vi "Trajectory Builder.vi"() -> ()   [LabVIEW 2019]
uses:
  Limits.ctl
  Command Stuff/Command Editor Info.ctl
  Command Stuff/Single Cmd Info.ctl
  <vilib>/picture/picture.llb/imagedata.ctl
  <vilib>/Utility/miscctls.llb/LVPositionTypeDef.ctl
  <vilib>/Utility/miscctls.llb/LVBoundsTypeDef.ctl
  Command Stuff/Availible Command systems for auto.ctl
  <vilib>/event_ctls.llb/lveventtype.ctl
  Globals.vi
panel:
  out "IRR":bool
  out "Trajectory Data":T1(array[cluster])
  in  "Reverse Path":bool
  in  "Robot Backwards":bool
  out "Picture":picture
  out "Duration (s)":dbl format="%#.4g"
  out "Distance (ft)":dbl format="%#.1g"
  in  "Instructions":string="Directions:\nUse mouse to ...\n    move robot position (rectangle with arrow)\n    rotate robot (red arrow)\n    move waypoints (numbered circles)\nClick in open space to add a waypoint\nShift click to delete a waypoint\nHover over a waypoint and use arrow keys to nudge\n\nTime slider and Play button will run robot along path to test for collisions.\n\nDirection and Destionation are folder selectors for files\n\nNew creates a new path at default location\n\nAppend creates a path using current path's position and heading.\n\nTo add a command, move robot using Time slider and double click Command in Palette.\n\nYou can modify command timing in the graph or Command Sequencer tree.\n\nEnable/disable a command by clicking on the enable column item.\n\nDelete a command by shift-clicking in the enable column.\n\nTo configure command parameters, Select the command name in the tree, Open Panel, enter parameters, and Inhale the parameters."
  out "WayPoints":cluster{"x":dbl, "y":dbl, "th":dbl}[](array[cluster]) {"th" format="%#_4g"}
  in  "Scale Factor":dbl=0.75
  out "Command Palette":picture
  in  "Cache":T5
  out "folder names":cluster{"name":string, "name":string}
  in  "Directory":bool
  in  "Tab Control":T6(tab)
  in  "Overrides":T7(array[cluster]) {"Angular Multiplier 2" step=5.0; "Angular Multiplier" step=5.0}
  in  "Allow Angles > 90":bool
  in  "Stoopid Overlap %":dbl min=0.0
  in  "Center Flip":bool
  in  "Snap to foot":bool
  in  "Angle Limiter":enum16{"90", "45", "15", "1"}(ring)=enum."15"
  in  "Snap robot to baseline":bool
  in  "Sample Period (s)":dbl=0.02 format="%#_6p"
  in  "Limits":T8={"Velocity (fps)"=6.0, "Accel (fps^2)"=15.0, "Jerk (fps^3)"=150.0, "StoopidFast (fps)"=6.0} {"StoopidFast (fps)" min=0.0; "Jerk (fps^3)" min=0.0 step=1.0; "Accel (fps^2)" min=0.0; "Velocity (fps)" min=0.0}
  in  "Conditions":T9 {"vFinal (fps)" min=0.0; "vInitial (fps)" min=0.0}
  in  "Unjank":bool
  in  "Turn Acceleration":bool=TRUE
  in  "Turn Deceleration":bool=TRUE
  in  "Hide Path":bool
  in  "Open Command":bool
  in  "Inhale":bool
  in  "Command Sequence":string(tree)
  in  "Projects":u16(ring) items=["2021 Robot.lvproj"]
  in  "Refresh":bool
  in  "Background":u16(ring) items=["IR Field", "Barrels", "Bounce", "Slalom", "Galactic Search A", "Galactic Search B"]
  in  "Robot Color":u32(colorbox)=14421504
  out "Field Size (ft)":cluster{"width":dbl, "height":dbl}={"width"=26.9167, "height"=35.2142} {"width" format="%#.1g"; "height" format="%#.1g"}
  in  "Robot Size (in)":cluster{"width":dbl, "height":dbl}={"width"=36.5, "height"=34.5}
  in  "Time (s)":dbl(slide) scale=0.0..3.62 scale format="%#.1g"
  in  "Play":bool
  in  "Sub Dir 2":u16(ring)
  in  "Sub Dir 1":u16(ring)
  out "fps":dbl[](graph)
  in  "Append":bool
  in  "Open":i32(listbox)
  in  "Filename":string
  in  "Save":bool
  in  "New":bool
  out "slalom":bool
  out "barrels":bool
  out "bounce":bool
  out "G-S B":bool
  out "G-S A":bool
  # "Command Palette"
  # "StupidFast makes each linear segment into a\nvelocity ramp to max speed"
  # "Nicotine"
  # "Interaction Options"
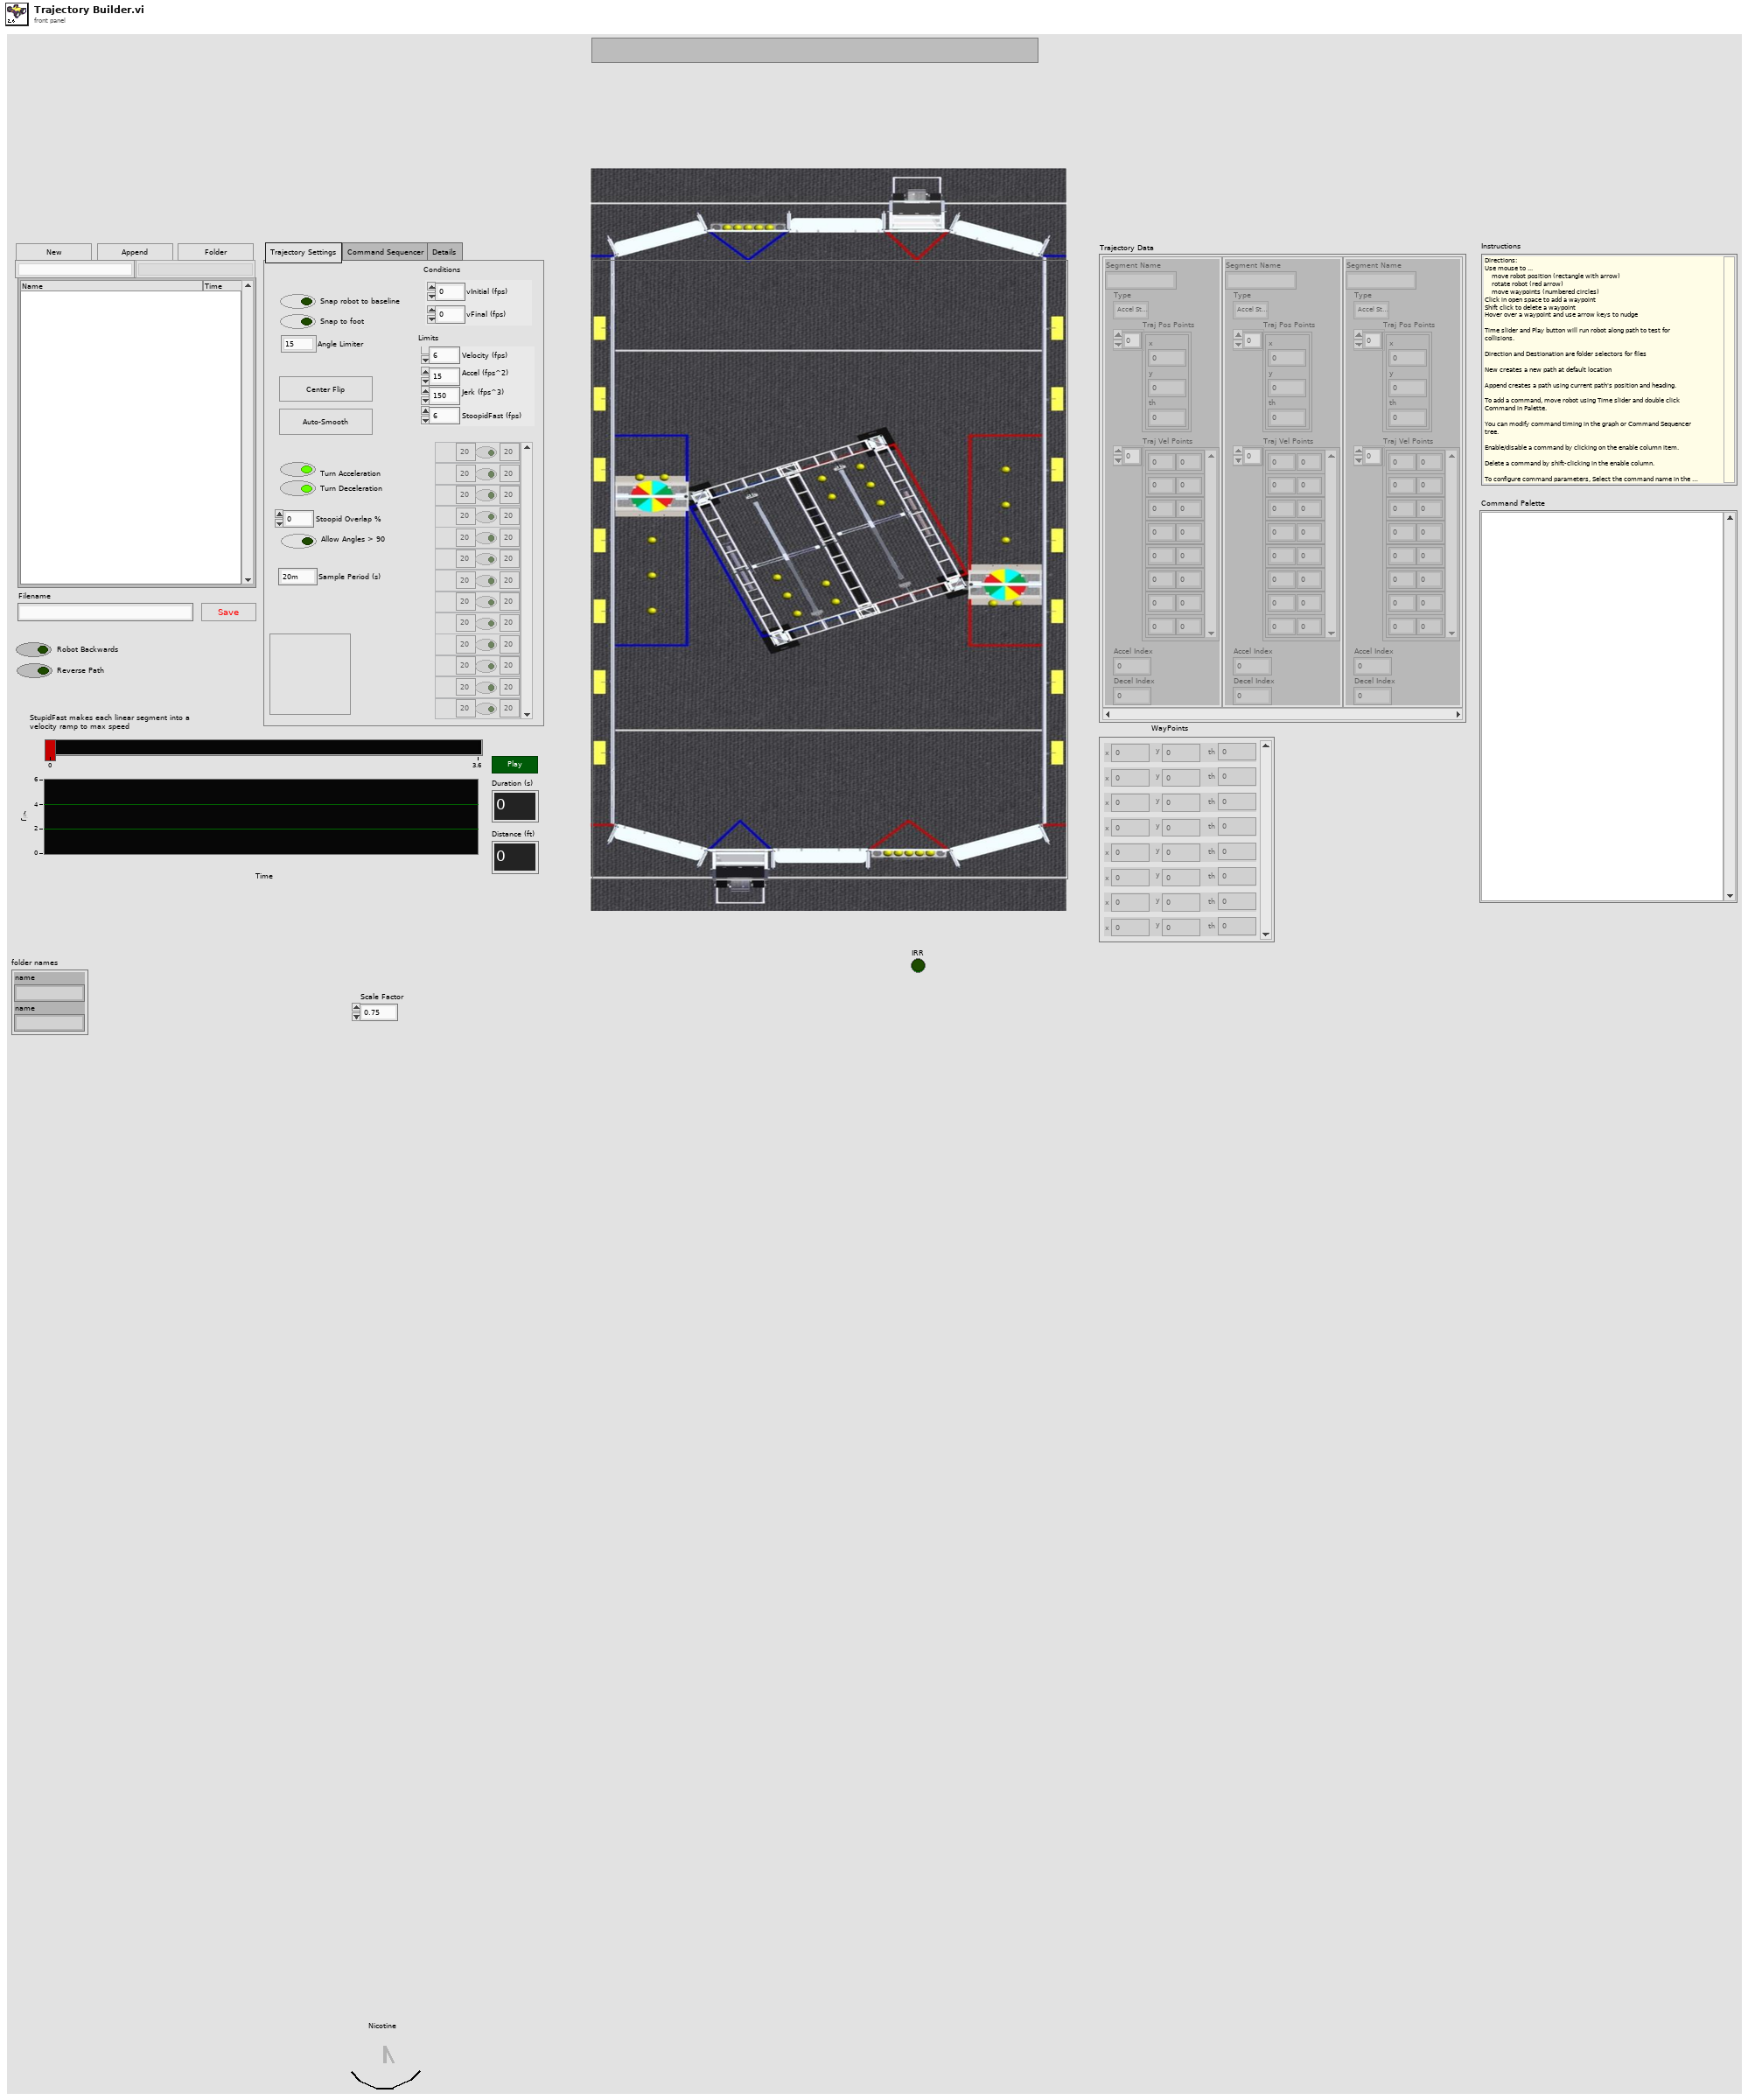
[diagram p1: front panel]
types:
  T1 = cluster{"Segment Name":string, "Type":enum16{"Accel Straight", "Const Straight", "Blend", "Circle"}, "Traj Pos Points":cluster{"x":dbl, "y":dbl, "th":dbl}[], "Traj Vel Points":cluster{"V":dbl, "th":dbl}[], "Accel Index":i32, "Decel Index":i32}[]
  T2 = typedef "Command Editor Info.ctl" = T3[]
  T3 = typedef "Single Cmd Info.ctl" = cluster{"Name":string, "CPTM.DataType":variant, "All Control Values Variant":cluster{"Name":string, "Variant Data":variant}[], "icon full":T4, "icon scaled":T4, "Path":path, "Subsystem Color":u32}
  T4 = typedef "imagedata.ctl" = cluster{"image type":i32, "image depth":i32, "image":u8[], "mask":u8[], "colors":u32[], "Rectangle":cluster{"left":i16, "top":i16, "right":i16, "bottom":i16}}
  T5 = cluster{"Filtered Command Info Out":T2, "2D Picture":picture}
  T6 = enum32{"Trajectory Settings", "Command Sequencer", "Details"}
  T7 = cluster{"Count":string, "Angular Multiplier":dbl, "1":bool, "Angular Multiplier 2":dbl}[]
  T8 = typedef "Limits.ctl" = cluster{"Velocity (fps)":dbl, "Accel (fps^2)":dbl, "Jerk (fps^3)":dbl, "StoopidFast (fps)":dbl}
  T9 = cluster{"vInitial (fps)":dbl, "vFinal (fps)":dbl}
  T10 = cluster{"Sample Period (s)":dbl, "Limits 2":T8, "Conditions":cluster{"vInitial (fps)":dbl, "vFinal (fps)":dbl}, "Angular \nAccelerations":cluster{string, "Angular Multiplier":dbl, "1":bool, "Angular Multiplier 2":dbl}[]}
  T11 = cluster{string, "Angular Multiplier":dbl, "1":bool, "Angular Multiplier 2":dbl}[]
  T12 = typedef "LVPositionTypeDef.ctl" = cluster{"Left":i32, "Top":i32}
  T13 = enum32{"Trajectory Settings", "Command Sequencer"}
  T14 = cluster{"Index":i32, "Pt Test Results":enum16{"Miss", "Rect Hit", "Arrow Hit"}}
  T15 = cluster{"Drag Object":cluster{"Index":i32, "x":dbl, "y":dbl}, "Hover Object":cluster{"Index":i32, "Pt Test Results":enum16{"Miss", "Rect Hit", "Arrow Hit"}}, "Filename":string}
  T16 = cluster{"Trajectory Data":cluster{"Segment Name":string, "Type":enum16{"Accel Straight", "Const Straight", "Blend", "Circle"}, "Traj Pos Points":cluster{"x":dbl, "y":dbl, "th":dbl}[], "Traj Vel Points":cluster{"V":dbl, "th":dbl}[], "Accel Index":i32, "Decel Index":i32}[], "Points":cluster{"x":dbl, "y":dbl, "th":dbl}[], "Cluster 2":cluster{"Sample Period (s)":dbl, "Limits 2":T8, "Conditions":cluster{"vInitial (fps)":dbl, "vFinal (fps)":dbl}, "Angular \nAccelerations":cluster{string, "Angular Multiplier":dbl, "1":bool, "Angular Multiplier 2":dbl}[]}, cluster{"Time (s)":dbl, T3, bool}[]}
  T17 = cluster{"Sample Period (s)":dbl, "Limits":cluster{"Velocity (fps)":dbl, "Accel (fps^2)":dbl, "Turn Accel (fps^2)":dbl, "Jerk (fps^3)":dbl}, "Conditions":cluster{"vInitial (fps)":dbl, "vFinal (fps)":dbl}, cluster{dbl[], bool[]}}
  T18 = cluster{"Sample Period (s)":dbl, "Limits":cluster{"Velocity (fps)":dbl, "Accel (fps^2)":dbl, "Jerk (fps^3)":dbl}, "Conditions":cluster{"vInitial (fps)":dbl, "vFinal (fps)":dbl}, " Acceleration Overrides":cluster{"Angular \nAccelerations":dbl[], "Accel Override Bools":bool[]}}
  T19 = typedef "LVBoundsTypeDef.ctl" = cluster{"Width":u32, "Height":u32}
  T20 = cluster{"Velocity":dbl, "Sample Time":dbl, "Accel":dbl}
  T21 = cluster{"Sample Period (s)":dbl, "Limits":cluster{"Velocity (fps)":dbl, "Acceleration (fps^2)":dbl, "Jerk (fps^3)":dbl}, "Conditions":cluster{"vInitial (fps)":dbl, "vFinal (fps)":dbl}}
  T22 = cluster{"Reverse Path":bool, "Robot Backwards":bool}
  T23 = cluster{"Sample Period (s)":dbl, "Limits 2":cluster{"Velocity (fps)":dbl, "Acceleration (fps^2)":dbl, "Jerk (fps^3)":dbl}, "Conditions":cluster{"vInitial (fps)":dbl, "vFinal (fps)":dbl}, " Acceleration Overrides":cluster{"Angular \nAccelerations":dbl[], "Accel Override Bools":bool[]}}
  T24 = cluster{"Sample Period (s)":dbl, "Limits":cluster{"Velocity (fps)":dbl, "Acceleration (fps^2)":dbl, "Jerk (fps^3)":dbl}, "Conditions":cluster{"vInitial (fps)":dbl, "vFinal (fps)":dbl}, "Min Rads":dbl[]}
  T25 = typedef "Availible Command systems for auto.ctl" = u16
  T26 = cluster{"Time into Path":dbl, "System":T25, "Item Selected?":bool, "System Selection":T25}[]
  T27 = cluster{"Sample Period (s)":dbl, "Limits 2":cluster{"Velocity (fps)":dbl, "Acceleration (fps^2)":dbl, "Jerk (fps^3)":dbl, "Stoopid Fast":dbl}, "Conditions":cluster{"vInitial (fps)":dbl, "vFinal (fps)":dbl}, " Acceleration Overrides":cluster{"Angular \nAccelerations":dbl[], "Accel Override Bools":bool[]}}
  T28 = typedef "lveventtype.ctl" = enum32{"Null", "Timeout", "Annotation Menu Selection", "Annotation Menu Selection?", "App Instance Close", "App Instance Close?", "Autoscale Range Change", "Bookmark Info Change", "Cell Edit", "Cell Edit?", "Cursor Grab", "Cursor Grab?", "Cursor Menu Selection", "Cursor Menu Selection?", "Cursor Move", "Cursor Release", "Data Change", "Direction Change", "Display State Change", "Drag Ended", "Drag Enter", "Drag Leave", "Drag Over", "Drag Source Update", "Drag Starting", "Drag Starting?", "Drop", "Exec State Change", "Key Down", "Key Down?", "Key Repeat", "Key Repeat?", "Key Up", "Listbox Double Click", "Menu Activation?", "Menu Selection (App)", "Menu Selection? (App)", "Menu Selection (User)", "Mouse Down", "Mouse Down?", "Mouse Enter", "Mouse Leave", "Mouse Move", "Mouse Up", "Mouse Wheel", "NI Security User Change (App)", "Pane Size", "Panel Close", "Panel Close?", "Panel Resize", "Plot Attribute Change", "Scale Range Change", "Shortcut Menu Activation?", "Shortcut Menu Selection (App)", "Shortcut Menu Selection? (App)", "Shortcut Menu Selection (User)", "Tree Double Click", "Tree Drag", "Tree Drag?", "Tree Drop", "Tree Drop?", "Tree Item Close", "Tree Item Close?", "Tree Item Open", "Tree Item Open?", "User Event", "Value Change"}
  T29 = enum32{"Invalid", "Standard", "Closed", "Hidden", "Minimized", "Maximized"}
  T30 = cluster{"Sample Period (s)":dbl, "Limits":T8, "Conditions":cluster{"vInitial (fps)":dbl, "vFinal (fps)":dbl}, "Overrides":cluster{"Count":string, "Angular Multiplier":dbl, "1":bool, "Angular Multiplier 2":dbl}[]}
  T31 = cluster{"width":dbl, "height":dbl, "width":dbl, "height":dbl}
  T32 = cluster{"Robot Backwards":bool, "Reverse Path":bool}
  T33 = cluster{"Sample Period (s)":dbl, "Limits":T8, "Conditions":cluster{"vInitial (fps)":dbl, "vFinal (fps)":dbl}, cluster{dbl[], bool[]}}
  T34 = cluster{"Trajectory Data":cluster{"Segment Name":string, "Type":enum16{"Accel Straight", "Const Straight", "Blend", "Circle"}, "Traj Pos Points":cluster{"x":dbl, "y":dbl, "th":dbl}[], "Traj Vel Points":cluster{"V":dbl, "th":dbl}[], "Accel Index":i32, "Decel Index":i32}[], "Updated Waypoints":cluster{"x":dbl, "y":dbl, "th":dbl}[], "Cluster 2":cluster{"Sample Period (s)":dbl, "Limits":T8, "Conditions":cluster{"vInitial (fps)":dbl, "vFinal (fps)":dbl}, "Overrides":cluster{"Count":string, "Angular Multiplier":dbl, "1":bool, "Angular Multiplier 2":dbl}[]}, cluster{"Time (s)":dbl, T3, bool}[]}
  T35 = cluster{"Velocity":dbl, "Accel":dbl, "Accel":dbl, "Velocity":dbl}
  T36 = cluster{"Velocity (fps)":dbl, "Acceleration (fps^2)":dbl, "Jerk (fps^3)":dbl}
  T37 = cluster{"Velocity (fps)":dbl, "Acceleration (fps^2)":dbl, "Jerk (fps^3)":dbl, "Velocity (fps)":dbl}
  T38 = cluster{string, "Angular Multiplier":dbl, bool, "Velocity (fps)":dbl}
  T39 = cluster{"Angular \nAccelerations":dbl[], "Accel Override Bools":bool[]}
  T40 = cluster{string, "Turn Accel":dbl, "Overtide":bool, "Velocity (fps)":dbl}[]
  T41 = cluster{"Velocity (fps)":dbl, "Acceleration (fps^2)":dbl, "Jerk (fps^3)":dbl, "Stoopid Fast":dbl}
  T42 = cluster{"Velocity (fps)":dbl, "Accel (fps^2)":dbl, "Turn Accel (fps^2)":dbl, "Jerk (fps^3)":dbl}
  T43 = cluster{"Sample Period (s)":dbl, cluster{"Velocity (fps)":dbl, "Accel (fps^2)":dbl, "Turn Accel (fps^2)":dbl, "Jerk (fps^3)":dbl}, "Conditions":cluster{"vInitial (fps)":dbl, "vFinal (fps)":dbl}, "Array":cluster{"Count":string, "Turn Accel":dbl, "Overtide":bool, "Velocity (fps)":dbl}[]}
  T44 = cluster{"Trajectory Data":cluster{"Segment Name":string, "Type":enum16{"Accel Straight", "Const Straight", "Blend", "Circle"}, "Traj Pos Points":cluster{"x":dbl, "y":dbl, "th":dbl}[], "Traj Vel Points":cluster{"V":dbl, "th":dbl}[], "Accel Index":i32, "Decel Index":i32}[], "Points":cluster{"x":dbl, "y":dbl, "th":dbl}[], cluster{"Sample Period (s)":dbl, cluster{"Velocity (fps)":dbl, "Accel (fps^2)":dbl, "Turn Accel (fps^2)":dbl, "Jerk (fps^3)":dbl}, "Conditions":cluster{"vInitial (fps)":dbl, "vFinal (fps)":dbl}, "Array":cluster{"Count":string, "Turn Accel":dbl, "Overtide":bool, "Velocity (fps)":dbl}[]}, cluster{"Time (s)":dbl, T3, bool}[]}
  T45 = typedef "LVPoint32TypeDef.ctl" = cluster{"Horizontal":i32, "Vertical":i32}
  T46 = cluster{"Shift":bool, "Ctrl":bool, "Alt":bool, "Cmd":bool, "Opt":bool}
  T47 = cluster{"Snap robot to baseline":bool, "Snap to foot":bool, "Angle Limiter":enum16{"90", "45", "15", "1"}}
  T48 = cluster{i32, "Pt Test Results":enum16{"Miss", "Rect Hit", "Arrow Hit"}}
  T49 = typedef "eventvkey.ctl" = enum16{"ASCII", "Enter", "Return", "Shift", "Ctrl", "Alt", "Cmd", "Opt", "Caps", "NumLock", "Clear", "Break", "Up", "Down", "Left", "Right", "Insert", "Delete", "Home", "End", "PageUp", "PageDown", "Escape", "Help", "Pause", "ScrollLock", "F1", "F2", "F3", "F4", "F5", "F6", "F7", "F8", "F9", "F10", "F11", "F12", "F13", "F14", "F15", "F16", "F17", "F18", "F19", "F20", "F21", "F22", "F23", "F24", "Play", "VolumeUp", "VolumeDown", "Mute", "Two Byte Char"}
  T50 = cluster{"Name":string, "CPTM.DataType":variant, "Get All Control Values Variant":cluster{"Name":string, "Variant Data":variant}[], "Color 256":T4, "Subsystem Color":u32}[]
  T51 = cluster{"Trajectory Data":cluster{"Segment Name":string, "Type":enum16{"Accel Straight", "Const Straight", "Blend", "Circle"}, "Traj Pos Points":cluster{"x":dbl, "y":dbl, "th":dbl}[], "Traj Vel Points":cluster{"V":dbl, "th":dbl}[], "Accel Index":i32, "Decel Index":i32}[], "Updated Waypoints":cluster{"x":dbl, "y":dbl, "th":dbl}[], cluster{"Sample Period (s)":dbl, "Limits":T8, "Conditions":cluster{"vInitial (fps)":dbl, "vFinal (fps)":dbl}, "Overrides":cluster{"Count":string, "Angular Multiplier":dbl, "1":bool, "Angular Multiplier 2":dbl}[]}, cluster{"Time (s)":dbl, T3, bool}[]}
  T52 = cluster{"Horizontal":dbl, "Vertical":dbl, "th":dbl}
  T53 = cluster{"Name":string, "Color":u32, "Style":i32, "Point Style":i32, "Name Visible":bool, "Allow Drag":bool, "Annotation Mode":i32, "Plot":i32, "Index":i32, "Position":cluster{"X":dbl, "Y":dbl}, "X Scale":i32, "Y Scale":u32, "Show Arrow":bool, "Lock Name":bool, "Plot Area":i32, "Label Offset":cluster{"X":dbl, "Y":dbl}}[]
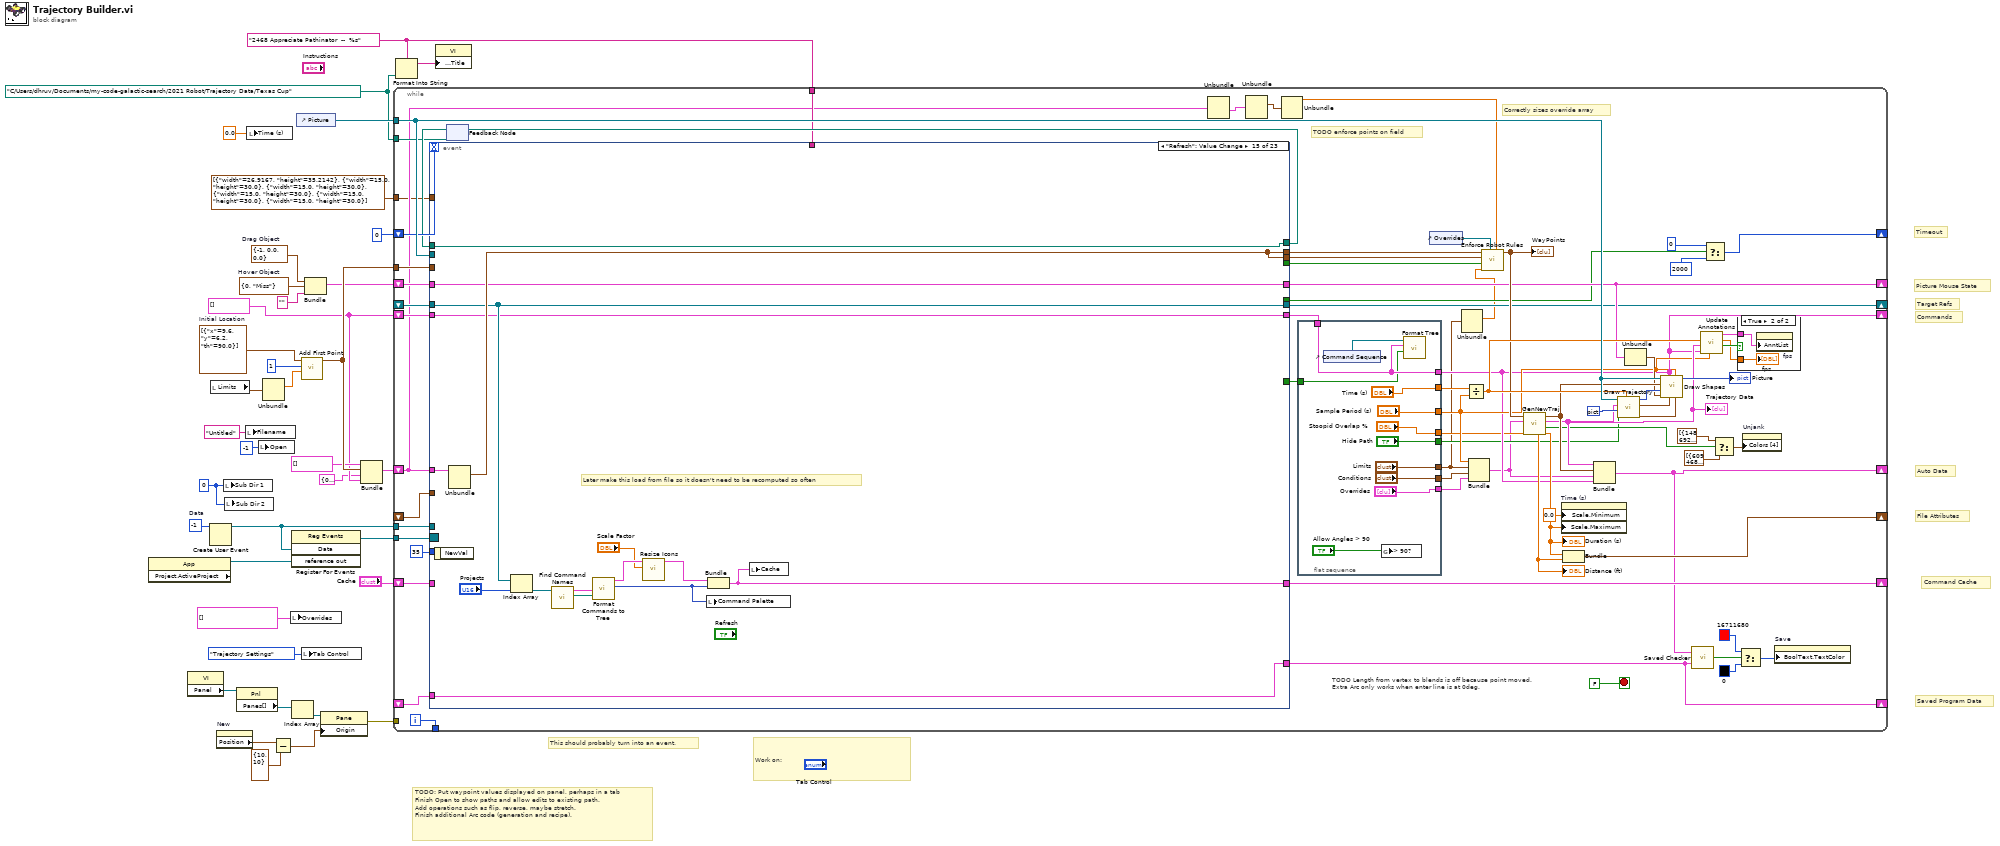
[diagram p0: block diagram]
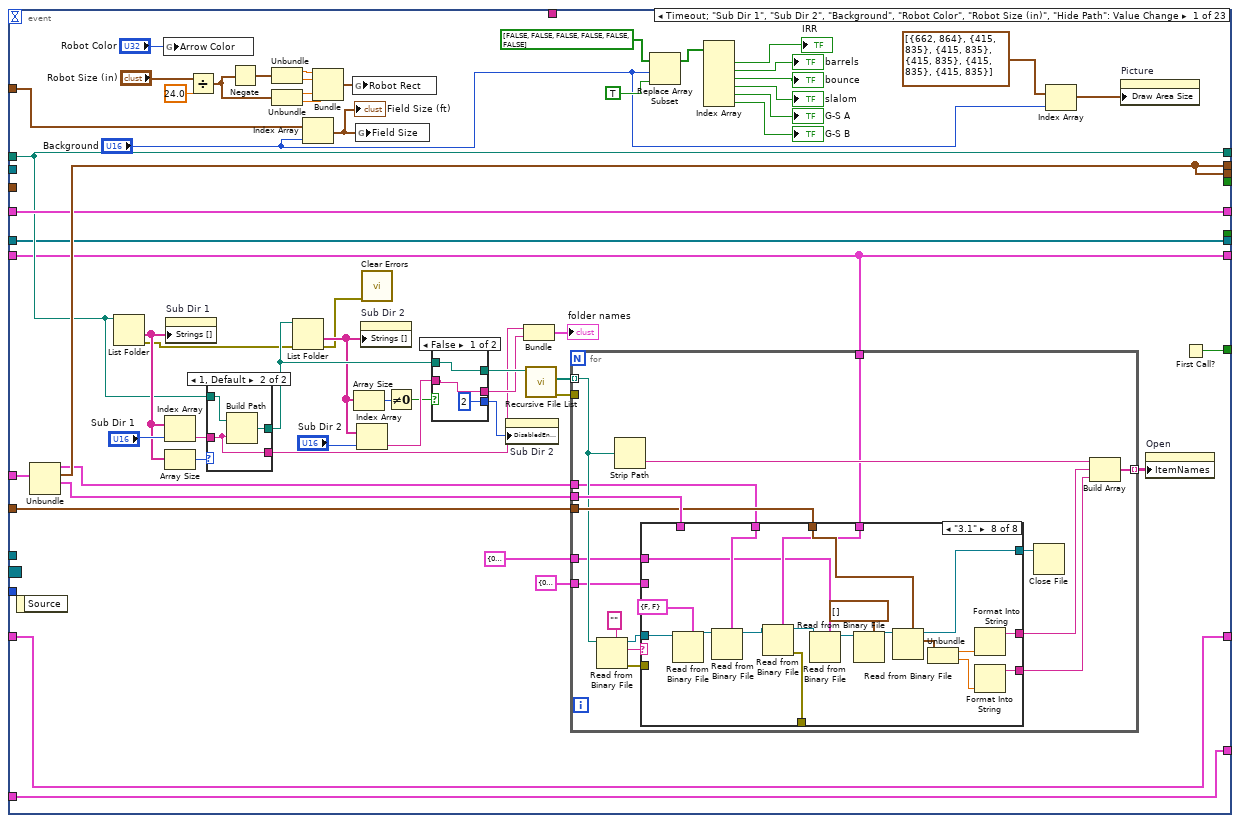
[diagram p3: hidden frame]
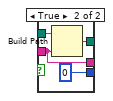
[diagram p5: hidden frame]
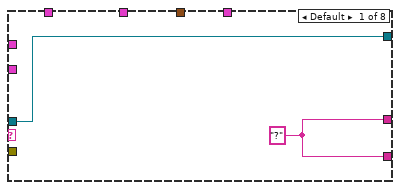
[diagram p6: hidden frame]
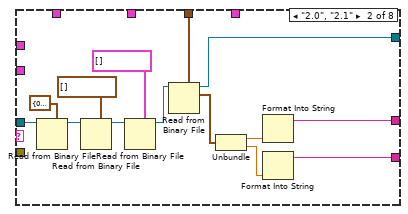
[diagram p7: hidden frame]
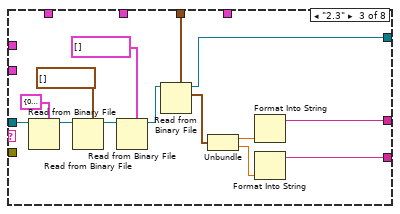
[diagram p8: hidden frame]
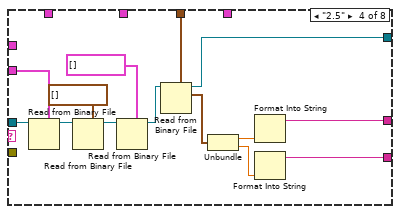
[diagram p9: hidden frame]
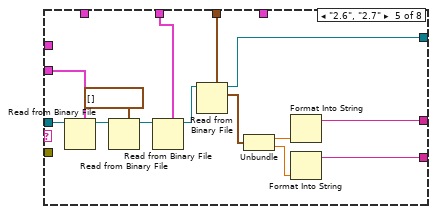
[diagram p10: hidden frame]
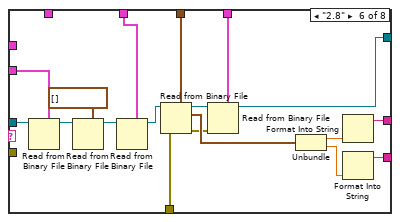
[diagram p11: hidden frame]
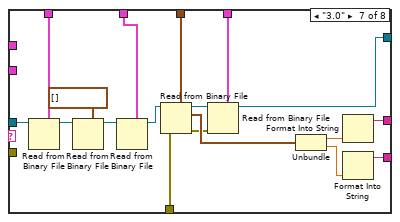
[diagram p12: hidden frame]
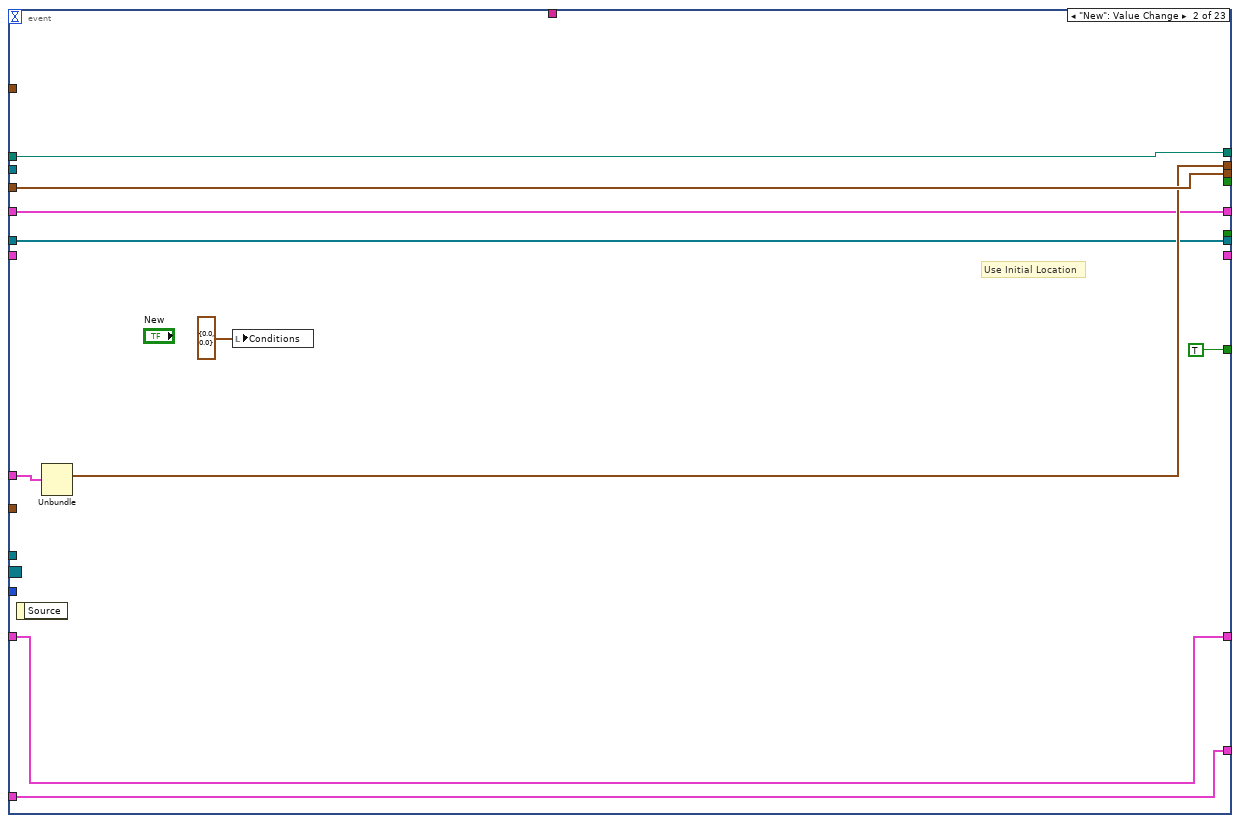
[diagram p13: hidden frame]
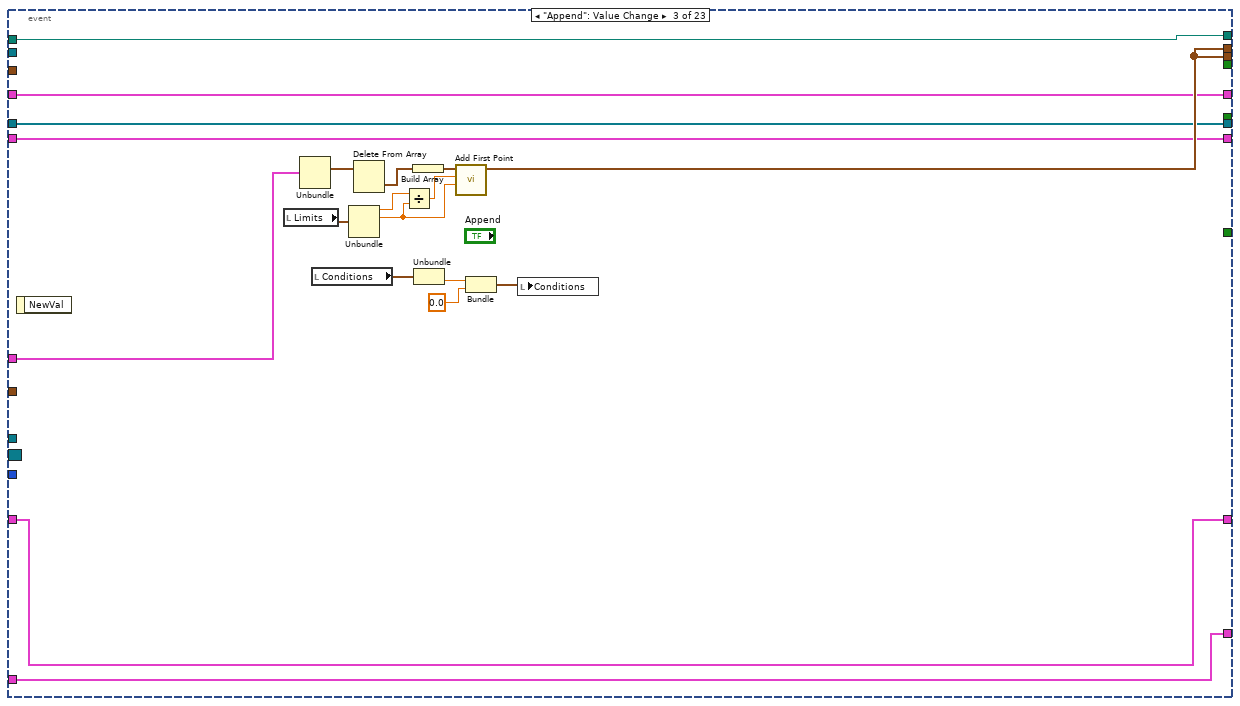
[diagram p14: hidden frame]
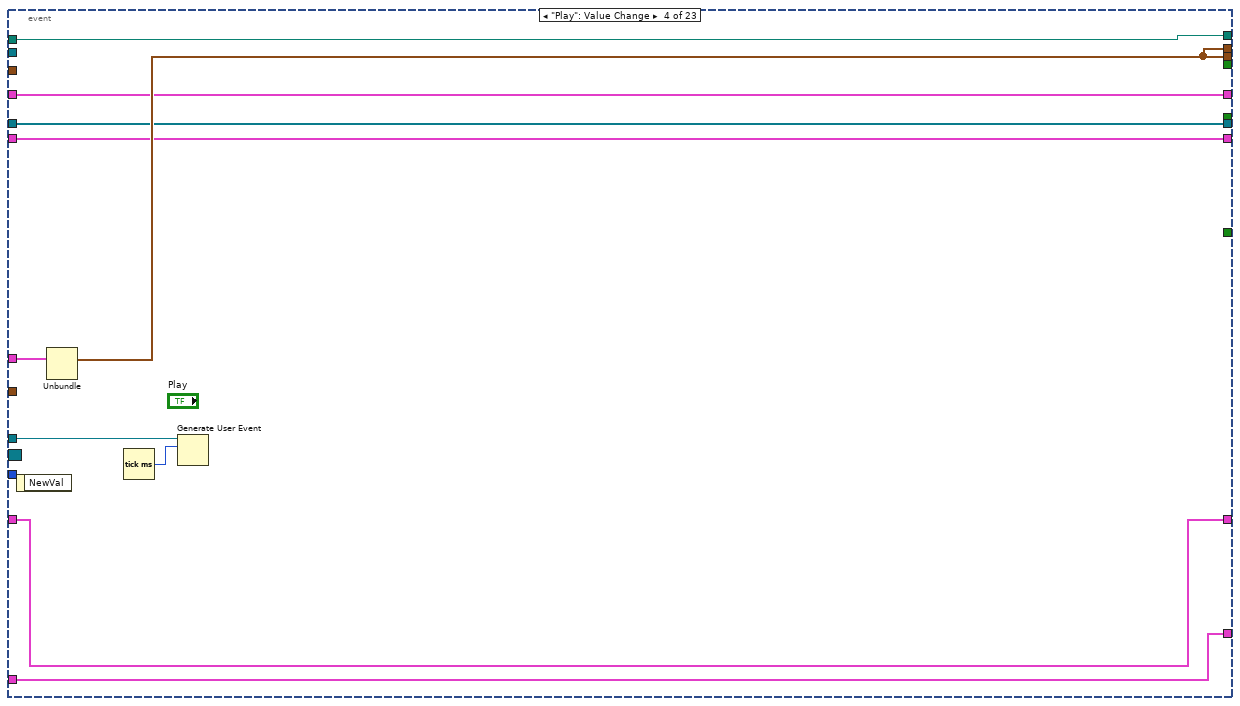
[diagram p15: hidden frame]
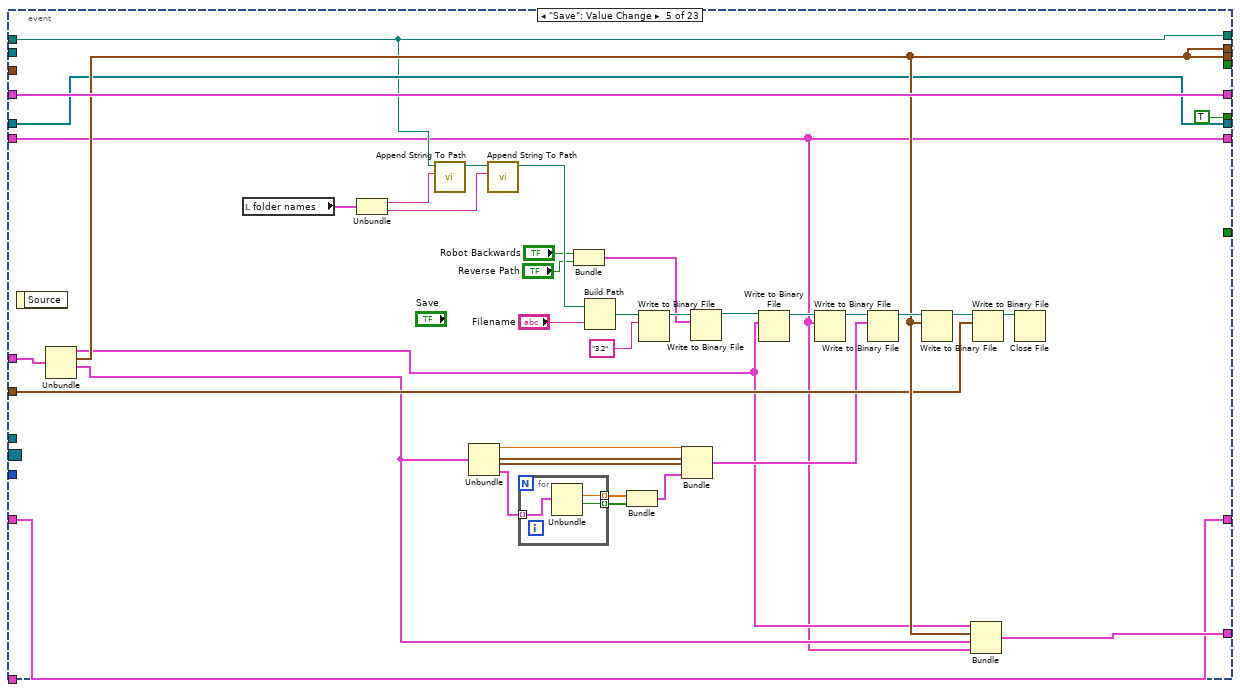
[diagram p16: hidden frame]
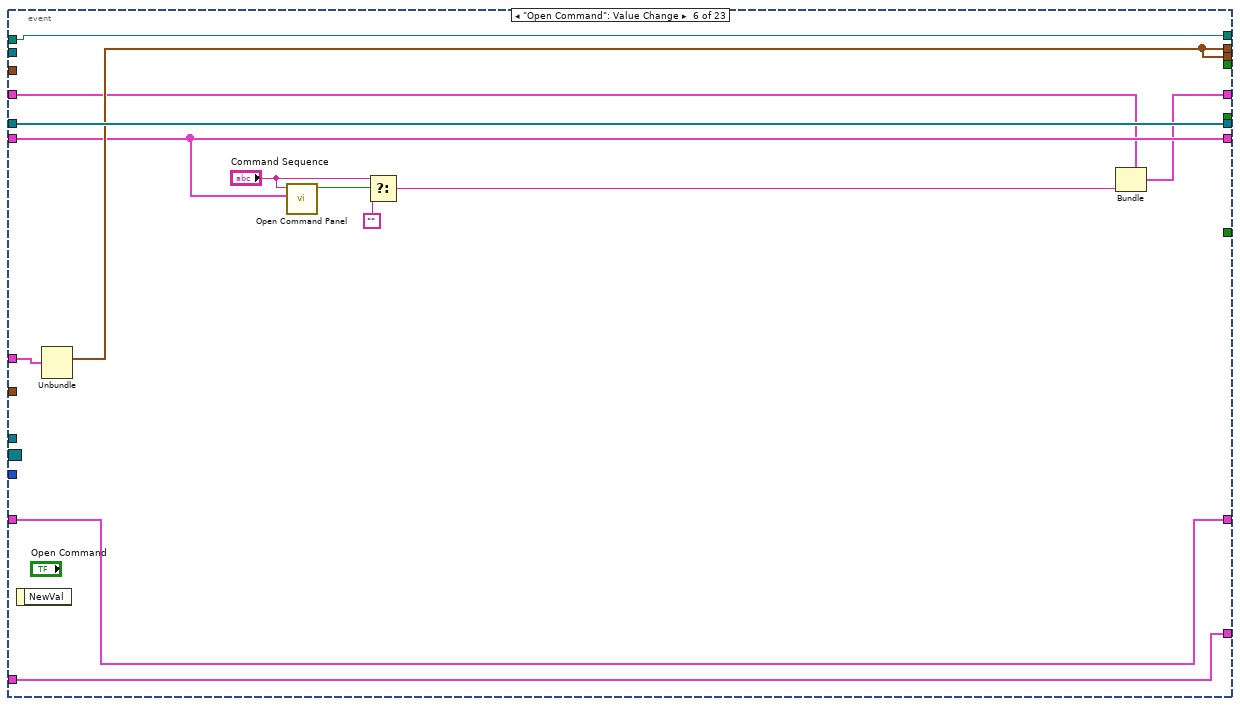
[diagram p17: hidden frame]
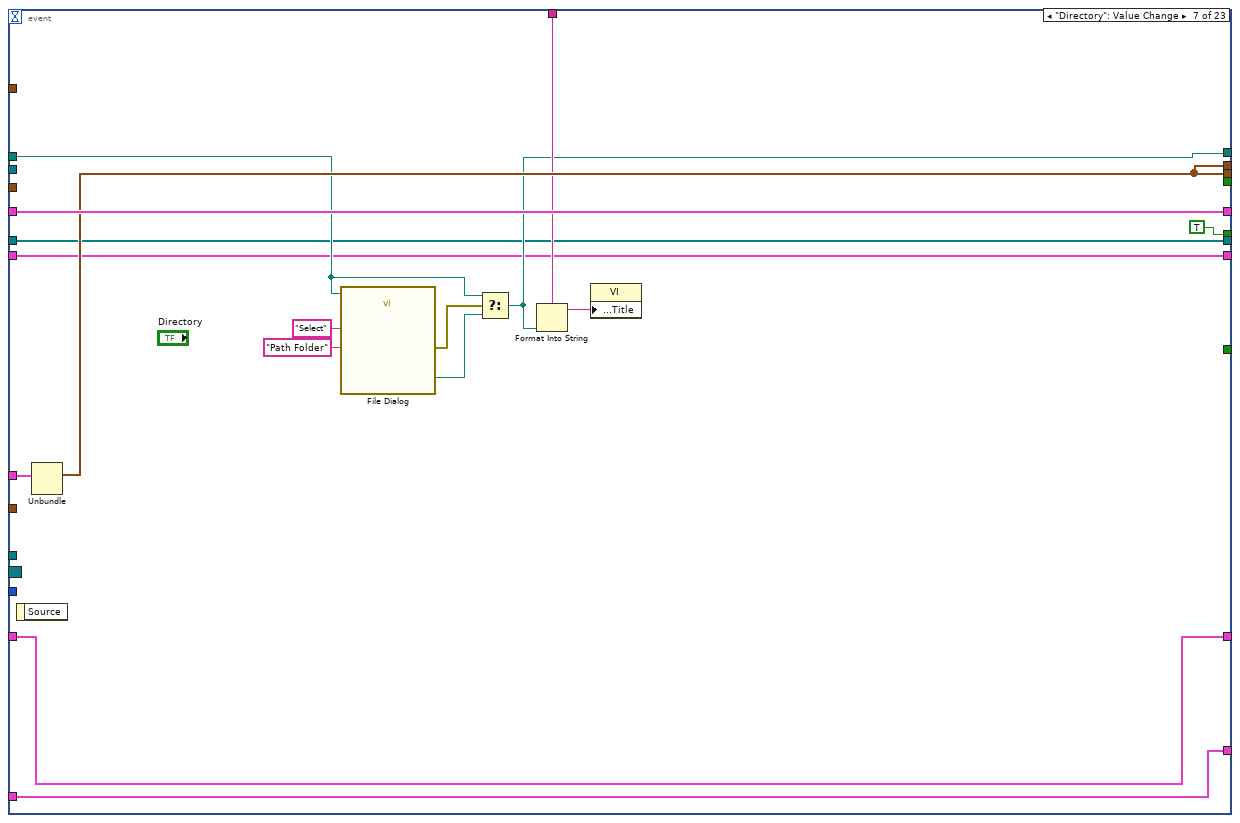
[diagram p18: hidden frame]
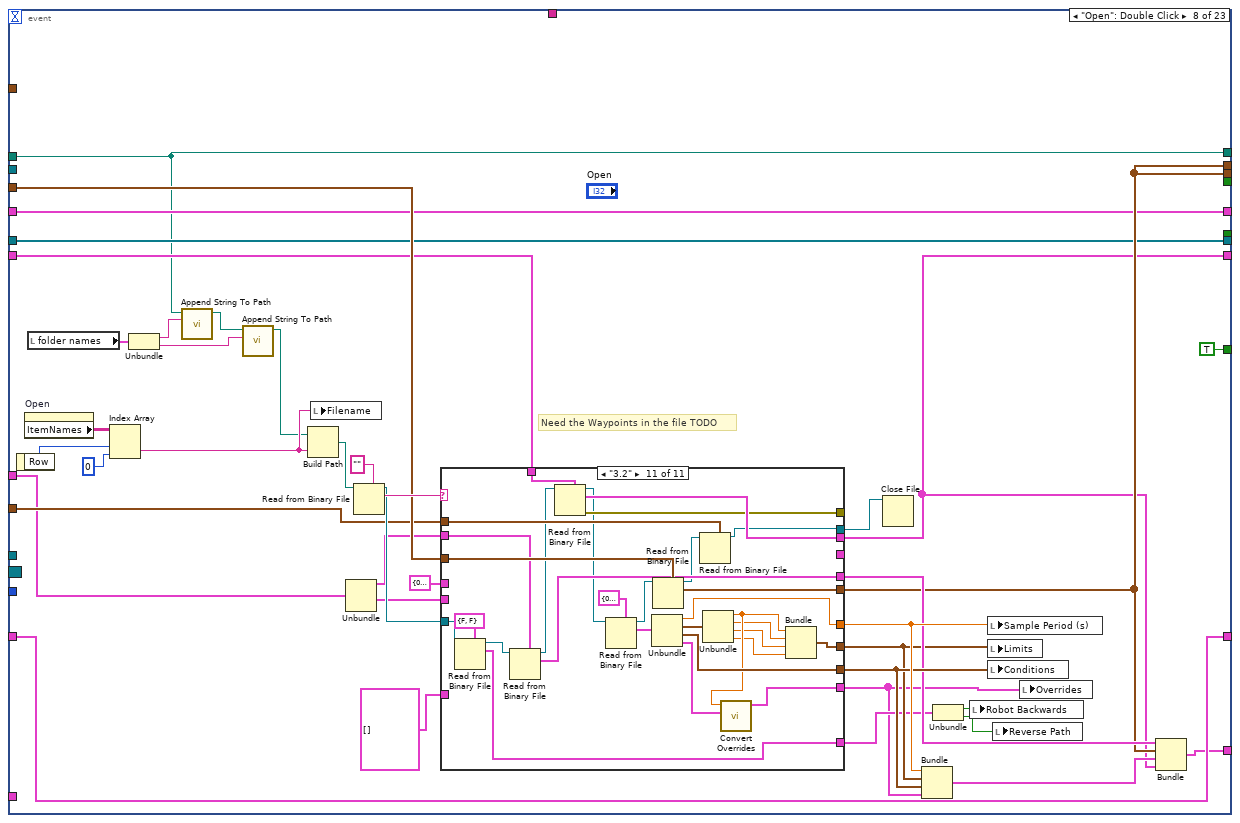
[diagram p19: hidden frame]
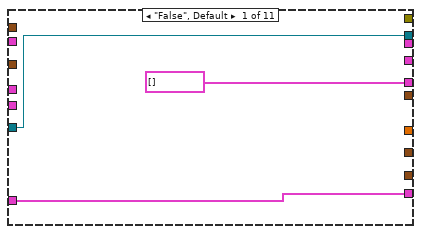
[diagram p20: hidden frame]
diagram:
  w3 = path "C:/Users/dhruv/Documents/my-code-galactic-search/2021 Robot/Trajectory Data/Texas Cup" ("Paths Location")
  w5 = cluster{"Time (s)":dbl, T3, bool}[] []
  w17 = 0 ("th")
  w18 = "2468 Appreciate Pathinator  --  %s" ("format string")
  w26 = -1  # Data
  w22 = T14 {"Index"=0, "Pt Test Results"=enum."Miss"}  # Hover Object
  w21 = cluster{"Index":i32, "x":dbl, "y":dbl} {"Index"=-1, "x"=0.0, "y"=0.0}  # Drag Object
  w35 = cluster{"x":dbl, "y":dbl, "th":dbl}[] [{"x"=9.6, "y"=6.2, "th"=90.0}]  # Initial Location
  # "Saved Program Data"
  # "Command Cache"
  # "File Attributes"
  # "Commands"
  # "Target Refs"
  # "Picture Mouse State"
  # "Auto Data"
  # "Timeout"
  # "This should probably turn into an event."
  # "Work on:"
  # "TODO: Put waypoint values displayed on panel, perhaps in a tab\nFinish Open to show paths and allow edits to existing path.\nAdd operations such as flip, reverse, maybe stretch.\nFinish additional Arc code (generation and recipe)."
  n1 = property class="App" props=["Project.ActiveProject"]() -> (reference out=w6:refnum<vi>)  [unwired: 2 in, 2 out]
  n2 = property class="VI"() -> ("Panel"=w14:refnum<vi>)  [unwired: 2 in, 2 out]
  n3 = Create User Event(user event datatype=w26) -> (user event=w27:refnum<user-event>)  [unwired: 1 in, 1 out]
  n4 = local read "Limits"() -> (w32:T8)
  n5 = property on="New" class="Bool"() -> ("Position"=w10:T12)  [unwired: 2 in, 2 out]
  n6 = local write "Sub Dir 1"(w17) -> ()
  n7 = local write "Sub Dir 2"(w17) -> ()
  n8 = property class="Pnl"(reference=w14) -> ("Panes[]"=w13:refnum<vi>[])  [unwired: 1 in, 2 out]
  n9 = local write "Filename"("Untitled" ("Filename")) -> ()
  n10 = local write "Time (s)"(0.0 ("Time")) -> ()
  n11 = local write "Open"(-1) -> ()
  n12 = Unbundle(w32) -> ("Accel (fps^2)"=w31:dbl)  [unwired: 3 out]
  n13 = Subtract(x=w10, y=T12 {"Left"=10, "Top"=10}) -> (x-y=w9:T12)
  n14 = local write "Overrides"(T11 [] ("Angular \nAccelerations")) -> ()
  n15 = register-events(w27, w6) -> (reference out=w28:refnum<event-registration>)  [unwired: 2 in, 1 out]
  n16 = Index Array(array=w13) -> (element=w12:refnum<vi>)  [unwired: 1 in]
  n17 = control-ref of="Picture"() -> (w37:refnum<vi>)
  n18 = call "Add First Point.vi"("Accel (f/s^2)"=w31, "Time (s)"=1 ("th"), "Initial Points"=w35) -> ("Points"=w25:cluster{"x":dbl, "y":dbl, "th":dbl}[])  [unwired: 8 in]
  n19 = local write "Tab Control"(T13."Trajectory Settings" ("Tab Control")) -> ()
  n20 = Bundle("Drag Object"=w21, "Hover Object"=w22, "Filename"="") -> (w20:T15)  [unwired: 1 in]
  n21 = property class="Pane"(reference=w12, "Origin"=w9) -> (error out=w8:errorcluster)  [unwired: 1 in, 1 out]
  n22 = Bundle("Trajectory Data"=T1 [], "Points"=w25, "Cluster 2"=T10 {"Sample Period (s)"=0.02, "Limits 2"={"Velocity (fps)"=6.0, "Accel (fps^2)"=32.0, "Jerk (fps^3)"=1500.0, "StoopidFast (fps)"=12.0}, "Conditions"={"vInitial (fps)"=0.0, "vFinal (fps)"=0.0}, "Angular \nAccelerations"=[]}, w5) -> (w24:T16)  [unwired: 1 in]
  n23 = while {
    tunnel: w25 -> [w109]
    tunnel: w37 -> [w108]
    shift-right: [w75] -> _
    shift-left: 0 -> [w102]
    shift-right: [w101] -> _
    shift-left: _ -> [w100]
    tunnel: w3 -> [w84]
    tunnel: w28 -> [w94]
    tunnel: w27 -> [w93]
    shift-right: [w91] -> _
    shift-left: _ -> [w92]
    shift-right: [w43] -> _
    shift-left: w24 -> [w52]
    shift-right: [w80] -> _
    shift-left: w20 -> [w81]
    tunnel: w18 -> [w78]
    shift-right: [w68] -> _
    shift-left: _ -> [w67]
    shift-right: [w65] -> _
    shift-left: "Cache" -> [w66]
    shift-right: [w58] -> _
    shift-left: w5 -> [w63]
    tunnel: w8 -> [_]
    tunnel: cluster{"width":dbl, "height":dbl}[] [{"width"=26.9167, "height"=35.2142}, {"width"=15.0, "height"=30.0}, {"width"=15.0, "height"=30.0}, {"width"=15.0, "height"=30.0}, {"width"=15.0, "height"=30.0}, {"width"=15.0, "height"=30.0}] -> [w49]
    tunnel: [w46] -> _
    i -> [w46]
    stop <- FALSE stop-if-true
    # "Correctly sizes override array"
    # "TODO Length from vertex to blends is off because point moved.\nExtra Arc only works when enter line is at 0deg."
    # "TODO enforce points on field"
    n24 = feedback #1(w84) -> (w85:path)
    n25 = event shown="[14] \"Refresh\": Value Change" {
      selector: w94 -> [_ _ _ _ _ _ _ _ _ _ _ _ _ _ _ _ _ _ _ _ _ _ _]
      dyn-events: _ -> [_ _ _ _ _ _ _ _ _ _ _ _ _ _ _ _ _ _ _ _ _ _ _]
      timeout: w102 -> [_ _ _ _ _ _ _ _ _ _ _ _ _ _ _ _ _ _ _ _ _ _ _]
      tunnel: [w163 w330 w348 w354 w390 w409 w426 w453 w724 w827 w871 w908 w932 w958 w977 w997 w1032 w1069 w1103 w1151 w1176 w1208 w1239] -> w99
      tunnel: w109 -> [_ w330 _ _ _ _ _ w462 _ _ _ _ _ _ _ _ _ _ _ _ _ _ _]
      tunnel: w108 -> [_ _ _ _ _ _ _ _ w723 w810 _ w895 _ _ _ _ _ _ _ _ _ _ _]
      tunnel: w85 -> [w161 w328 w337 w359 w384 w413 w420 w441 w721 w821 w866 w909 w948 w961 w979 w1001 w1036 w1075 w1108 w1155 w1181 w1213 w1244]
      tunnel: [w163 w325 w348 w354 w390 w409 w426 w453 w718 w818 w862 w893 w932 w958 w977 w997 w1032 w1069 w1103 w1151 w1176 w1208 w1239] -> w98
      tunnel: w100 -> [w179 _ _ _ w386 _ _ w460 _ _ _ _ _ _ _ _ _ _ _ _ _ _ _]
      tunnel: [_ _ _ _ _ _ _ _ _ _ TRUE ("Flip Over Center") _ _ _ _ _ _ _ _ _ _ _ _] -> w97
      tunnel: [w161 w328 w337 w359 w384 w413 w418 w441 w721 w821 w866 w909 w948 w961 w979 w1001 w1036 w1075 w1108 w1155 w1181 w1213 w1244] -> w86
      tunnel: w93 -> [_ _ _ w358 _ _ _ _ _ _ _ _ w947 _ _ _ _ _ _ _ _ _ _]
      tunnel: [w172 w327 w338 w357 w393 w412 w428 w430 w720 w820 w865 w896 w944 w960 w980 w1000 w1035 w1074 w1107 w1154 w1180 w1212 w1243] -> w91
      tunnel: w92 -> [w172 w327 w338 w357 _ w412 w428 _ w720 w820 w865 w896 w944 w960 w980 w1000 w1035 w1074 w1107 w1154 w1180 w1212 w1243]
      tunnel: w52 -> [w165 w326 w336 w355 w392 w410 w427 w452 w719 w819 w863 w894 w933 w959 w978 w998 w1033 w1071 w1104 w1152 w1177 w1209 w1240]
      tunnel: w81 -> [w162 w324 w334 w353 w391 w406 w429 w450 w715 w811 w861 w891 w931 w957 w976 w996 w1031 w1073 w1106 w1137 w1179 w1211 w1242]
      tunnel: [w162 w324 w334 w353 w391 w407 w429 w450 w717 w815 w861 w891 w931 w957 w976 w996 w1031 w1073 w1106 w1138 w1179 w1211 w1242] -> w80
      tunnel: w78 -> [_ _ _ _ _ _ w423 _ _ _ _ _ _ _ _ _ _ _ _ _ _ _ _]
      tunnel: [_ _ _ _ TRUE _ TRUE _ _ _ _ _ _ _ _ _ _ _ _ _ _ _ _] -> w74
      tunnel: [w158 w322 w333 w352 w388 w411 w417 w447 w711 w813 w858 w889 w930 w955 w975 w999 w1034 w1072 w1105 w1153 w1178 w1210 w1241] -> w68
      tunnel: w67 -> [w158 w322 w333 w352 w388 w411 w417 w447 w711 w813 w858 w889 w930 w954 w975 w999 w1034 w1072 w1105 w1153 w1178 w1210 w1241]
      tunnel: w66 -> [w155 w323 w332 w351 w387 w401 w416 w446 w713 w812 w857 w888 w929 w953 _ w981 w1023 w1062 w1088 w1135 w1161 w1199 w1226]
      tunnel: [w155 w323 w332 w351 w387 w401 w416 w446 w713 w812 w857 w888 w929 w953 w969 w981 w1023 w1062 w1088 w1135 w1161 w1199 w1226] -> w65
      tunnel: 35 -> [_ _ _ _ _ _ _ _ _ _ _ _ _ _ _ _ _ _ _ _ _ w1201 w1235]
      tunnel: w63 -> [w153 _ w331 w350 w360 w408 w414 w444 w712 w809 w856 w887 w928 w952 w968 w982 w1025 w1067 w1091 w1140 w1164 w1200 w1228]
      tunnel: [w153 _ w331 w350 w360 w408 w414 w437 w712 w809 w856 w887 w928 w952 w968 w982 w1026 w1068 w1089 w1140 w1165 w1200 w1229] -> w62
      tunnel: [w152 TRUE _ _ _ _ _ TRUE _ _ _ _ _ _ _ w989 w1024 TRUE w1090 _ w1163 _ TRUE] -> w61
      tunnel: w49 -> [w129 _ _ _ _ _ _ _ _ _ _ _ _ _ _ _ _ _ _ _ _ _ _]
      event Timeout; "Sub Dir 1", "Sub Dir 2", "Background", "Robot Color", "Robot Size (in)", "Hide Path": Value Change {
        n26 = event-data() -> ()  [unwired: 1 in, 1 out]
        n27 = Unbundle(w165) -> ("Trajectory Data"=w154:T1, "Updated Waypoints"=w163:cluster{"x":dbl, "y":dbl, "th":dbl}[], "Cluster 2"=w164:T30)  [unwired: 1 out]
        n28 = List Folder(path=w161) -> (folder names=w168:string[], error out=w157:errorcluster)  [unwired: 3 in, 2 out]
        n29 = global write "Globals.vi" "Arrow Color"("Robot Color") -> ()
        n30 = Index Array(array=w168, index="Sub Dir 1") -> (element=w169:string)
        n31 = Array Size(array=w168) -> (size(s)=w166:i32)
        n32 = property on="Sub Dir 1" class="Ring (strict)"("Strings []"=w168) -> ()  [unwired: 2 in, 2 out]
        n33 = Divide(x="Robot Size (in)", y=24.0 ("width")) -> (x/y=w146:cluster{"width":dbl, "height":dbl})
        n34 = case shown="1, Default" w166 {
          tunnel: w161 -> [w183 w186]
          tunnel: [w183 w185] -> w170
          tunnel: w169 -> [w182 w184]
          tunnel: [w182 w184] -> w150
          frame 0 {
          }
          frame 1, Default {
            n35 = Build Path(base path=w186, name or relative path=w184) -> (appended path=w185:path)
          }
        }
        n36 = Negate(x=w146) -> (-x=w147:cluster{"width":dbl, "height":dbl})
        n37 = Unbundle(w147) -> ("width"=w145:dbl, "height"=w144:dbl)
        n38 = Unbundle(w146) -> ("width"=w143:dbl, "height"=w142:dbl)
        n39 = List Folder(path=w170, error in=w157) -> (folder names=w167:string[], error out=w156:errorcluster)  [unwired: 2 in, 2 out]
        n40 = Index Array(array=w129, index="Background") -> (element=w128:cluster{"width":dbl, "height":dbl})
        "Field Size (ft)" <- w128
        n41 = Bundle("width"=w145, "height"=w144, "width"=w143, "height"=w142) -> (w141:T31)  [unwired: 1 in]
        n42 = global write "Globals.vi" "Robot Rect"(w141) -> ()
        n43 = Array Size(array=w167) -> (size(s)=w171:i32)
        n44 = global write "Globals.vi" "Field Size"(w128) -> ()
        n45 = Index Array(array=w167, index="Sub Dir 2") -> (element=w175:string)
        n46 = property on="Sub Dir 2" class="Ring (strict)"("Strings []"=w167) -> ()  [unwired: 2 in, 2 out]
        n47 = call <vilib>:"Clear Errors.vi"("error in (no error)"=w156) -> ()  [unwired: 5 in, 2 out]
        n48 = Not Equal To 0?(x=w171) -> (x != 0?=w174:bool)
        n49 = case shown="False" w174 {
          tunnel: w170 -> [w189 w193]
          tunnel: [w189 w192] -> w160
          tunnel: w175 -> [w187 w190]
          tunnel: [2 0] -> w173
          tunnel: [w187 w190] -> w151
          frame False {
          }
          frame True {
            n50 = Build Path(base path=w193, name or relative path=w190) -> (appended path=w192:path)
          }
        }
        n51 = property on="Sub Dir 2" class="Ring (strict)"("DisabledEnum"=w173) -> ()  [unwired: 2 in, 2 out]
        n52 = Bundle(w150, w151) -> (→"folder names":cluster{string, string})  [unwired: 1 in]
        n53 = call <vilib>:"Recursive File List.vi"("Folder Path"=w160) -> ("error out"=w178:errorcluster, "All Files in Dir"=w181:path[])  [unwired: 6 in, 3 out]
        n54 = for {
          tunnel: w181 -> [w199] mode=indexing
          tunnel: [w209] -> w180 mode=indexing
          tunnel: w164 -> [w204]
          tunnel: w179 -> [w203]
          tunnel: w178 -> [_]
          tunnel: w154 -> [w198]
          tunnel: w153 -> [w197]
          tunnel: T18 {"Sample Period (s)"=0.0, "Limits"={"Velocity (fps)"=0.0, "Accel (fps^2)"=0.0, "Jerk (fps^3)"=0.0}, "Conditions"={"vInitial (fps)"=0.0, "vFinal (fps)"=0.0}, " Acceleration Overrides"={"Angular \nAccelerations"=[], "Accel Override Bools"=[]}} ("Cluster") -> [w196]
          tunnel: T17 {"Sample Period (s)"=0.0, "Limits"={"Velocity (fps)"=0.0, "Accel (fps^2)"=0.0, "Turn Accel (fps^2)"=15.0, "Jerk (fps^3)"=0.0}, "Conditions"={"vInitial (fps)"=0.0, "vFinal (fps)"=0.0}, {[], []}} ("Cluster 2") -> [w194]
          n55 = Read from Binary File(5:"", 11:w199) -> (0:w195:errorcluster, 2:w207:string, 3:w206:refnum<file>)  [unwired: 4 in, 1 out]
          n56 = Strip Path(path=w199) -> (name=w200:string)  [unwired: 1 out]
          n57 = case shown="\"3.1\"" w207 {
            tunnel: [w211 w225 w239 w253 w267 w284 w301 w320] -> w202
            tunnel: [w211 w224 w238 w252 w266 w283 w300 w319] -> w201
            tunnel: w206 -> [w210 w223 w237 w251 w265 w282 w299 w309]
            tunnel: [w210 w219 w233 w247 w261 w271 w288 w307] -> w205
            tunnel: w204 -> [_ _ _ _ _ _ w285 _]
            tunnel: w203 -> [_ w218 w232 w246 w260 w278 w295 w317]
            tunnel: w198 -> [_ _ _ _ w255 w273 w290 w308]
            tunnel: w197 -> [_ _ _ _ _ w270 w287 w312]
            tunnel: [_ _ _ _ _ w269 w286 w311] -> _
            tunnel: w196 -> [_ _ _ w240 w254 w268 _ _]
            tunnel: w195 -> [_ _ _ _ _ _ _ _]
            tunnel: w194 -> [_ _ _ _ _ _ _ w302]
            frame Default {
              w211 = "?"
            }
            frame "2.0", "2.1" {
              n58 = Read from Binary File(5:T20 {"Velocity"=0.0, "Sample Time"=0.0, "Accel"=0.0}, 11:w223) -> (3:w222:refnum<file>)  [unwired: 4 in, 3 out]
              n59 = Read from Binary File(5:cluster{"x":dbl, "y":dbl, "th":dbl}[] [] ("Points"), 11:w222) -> (3:w221:refnum<file>)  [unwired: 4 in, 3 out]
              n60 = Read from Binary File(5:T1 [] ("Trajectory Data"), 11:w221) -> (3:w220:refnum<file>)  [unwired: 4 in, 3 out]
              n61 = Read from Binary File(5:w218, 11:w220) -> (2:w213:cluster{"Time (s)":dbl, "Distance (ft)":dbl}, 3:w219:refnum<file>)  [unwired: 4 in, 2 out]
              n62 = Unbundle(w213) -> ("Time (s)"=w217:dbl, "Distance (ft)"=w216:dbl)
              n63 = Format Into String(w217) -> (resulting string=w225:string)  [unwired: 3 in, 1 out]
              n64 = Format Into String(w216) -> (resulting string=w224:string)  [unwired: 3 in, 1 out]
            }
            frame "2.3" {
              n65 = Read from Binary File(5:T21 {"Sample Period (s)"=0.0, "Limits"={"Velocity (fps)"=0.0, "Acceleration (fps^2)"=0.0, "Jerk (fps^3)"=0.0}, "Conditions"={"vInitial (fps)"=0.0, "vFinal (fps)"=0.0}}, 11:w237) -> (3:w236:refnum<file>)  [unwired: 4 in, 3 out]
              n66 = Read from Binary File(5:cluster{"x":dbl, "y":dbl, "th":dbl}[] [] ("Points"), 11:w236) -> (3:w235:refnum<file>)  [unwired: 4 in, 3 out]
              n67 = Read from Binary File(5:T1 [] ("Trajectory Data"), 11:w235) -> (3:w234:refnum<file>)  [unwired: 4 in, 3 out]
              n68 = Read from Binary File(5:w232, 11:w234) -> (2:w227:cluster{"Time (s)":dbl, "Distance (ft)":dbl}, 3:w233:refnum<file>)  [unwired: 4 in, 2 out]
              n69 = Unbundle(w227) -> ("Time (s)"=w231:dbl, "Distance (ft)"=w230:dbl)
              n70 = Format Into String(w231) -> (resulting string=w239:string)  [unwired: 3 in, 1 out]
              n71 = Format Into String(w230) -> (resulting string=w238:string)  [unwired: 3 in, 1 out]
            }
            frame "2.5" {
              n72 = Read from Binary File(5:w240, 11:w251) -> (3:w250:refnum<file>)  [unwired: 4 in, 3 out]
              n73 = Read from Binary File(5:cluster{"x":dbl, "y":dbl, "th":dbl}[] [] ("Points"), 11:w250) -> (3:w249:refnum<file>)  [unwired: 4 in, 3 out]
              n74 = Read from Binary File(5:T1 [] ("Trajectory Data"), 11:w249) -> (3:w248:refnum<file>)  [unwired: 4 in, 3 out]
              n75 = Read from Binary File(5:w246, 11:w248) -> (2:w241:cluster{"Time (s)":dbl, "Distance (ft)":dbl}, 3:w247:refnum<file>)  [unwired: 4 in, 2 out]
              n76 = Unbundle(w241) -> ("Time (s)"=w245:dbl, "Distance (ft)"=w244:dbl)
              n77 = Format Into String(w245) -> (resulting string=w253:string)  [unwired: 3 in, 1 out]
              n78 = Format Into String(w244) -> (resulting string=w252:string)  [unwired: 3 in, 1 out]
            }
            frame "2.6", "2.7" {
              n79 = Read from Binary File(5:w254, 11:w265) -> (3:w264:refnum<file>)  [unwired: 4 in, 3 out]
              n80 = Read from Binary File(5:cluster{"x":dbl, "y":dbl, "th":dbl}[] [] ("Points"), 11:w264) -> (3:w263:refnum<file>)  [unwired: 4 in, 3 out]
              n81 = Read from Binary File(5:w255, 11:w263) -> (3:w262:refnum<file>)  [unwired: 4 in, 3 out]
              n82 = Read from Binary File(5:w260, 11:w262) -> (2:w256:cluster{"Time (s)":dbl, "Distance (ft)":dbl}, 3:w261:refnum<file>)  [unwired: 4 in, 2 out]
              n83 = Unbundle(w256) -> ("Time (s)"=w259:dbl, "Distance (ft)"=w258:dbl)
              n84 = Format Into String(w259) -> (resulting string=w267:string)  [unwired: 3 in, 1 out]
              n85 = Format Into String(w258) -> (resulting string=w266:string)  [unwired: 3 in, 1 out]
            }
            frame "2.8" {
              n86 = Read from Binary File(5:w268, 11:w282) -> (3:w281:refnum<file>)  [unwired: 4 in, 3 out]
              n87 = Read from Binary File(5:cluster{"x":dbl, "y":dbl, "th":dbl}[] [] ("Points"), 11:w281) -> (3:w280:refnum<file>)  [unwired: 4 in, 3 out]
              n88 = Read from Binary File(5:w273, 11:w280) -> (3:w279:refnum<file>)  [unwired: 4 in, 3 out]
              n89 = Read from Binary File(5:w278, 11:w279) -> (2:w274:cluster{"Time (s)":dbl, "Distance (ft)":dbl}, 3:w272:refnum<file>)  [unwired: 4 in, 2 out]
              n90 = Read from Binary File(5:w270, 11:w272) -> (0:w269:errorcluster, 3:w271:refnum<file>)  [unwired: 4 in, 2 out]
              n91 = Unbundle(w274) -> ("Time (s)"=w277:dbl, "Distance (ft)"=w276:dbl)
              n92 = Format Into String(w277) -> (resulting string=w284:string)  [unwired: 3 in, 1 out]
              n93 = Format Into String(w276) -> (resulting string=w283:string)  [unwired: 3 in, 1 out]
            }
            frame "3.0" {
              n94 = Read from Binary File(5:w285, 11:w299) -> (3:w298:refnum<file>)  [unwired: 4 in, 3 out]
              n95 = Read from Binary File(5:cluster{"x":dbl, "y":dbl, "th":dbl}[] [] ("Points"), 11:w298) -> (3:w297:refnum<file>)  [unwired: 4 in, 3 out]
              n96 = Read from Binary File(5:w290, 11:w297) -> (3:w296:refnum<file>)  [unwired: 4 in, 3 out]
              n97 = Read from Binary File(5:w295, 11:w296) -> (2:w291:cluster{"Time (s)":dbl, "Distance (ft)":dbl}, 3:w289:refnum<file>)  [unwired: 4 in, 2 out]
              n98 = Read from Binary File(5:w287, 11:w289) -> (0:w286:errorcluster, 3:w288:refnum<file>)  [unwired: 4 in, 2 out]
              n99 = Unbundle(w291) -> ("Time (s)"=w294:dbl, "Distance (ft)"=w293:dbl)
              n100 = Format Into String(w294) -> (resulting string=w301:string)  [unwired: 3 in, 1 out]
              n101 = Format Into String(w293) -> (resulting string=w300:string)  [unwired: 3 in, 1 out]
            }
            frame "3.1" {
              n102 = Read from Binary File(5:T22 {"Reverse Path"=FALSE, "Robot Backwards"=FALSE} ("Cluster"), 11:w309) -> (3:w303:refnum<file>)  [unwired: 4 in, 3 out]
              n103 = Read from Binary File(5:w308, 11:w303) -> (3:w306:refnum<file>)  [unwired: 4 in, 3 out]
              n104 = Read from Binary File(5:w312, 11:w306) -> (0:w311:errorcluster, 3:w305:refnum<file>)  [unwired: 4 in, 2 out]
              n105 = Read from Binary File(5:w302, 11:w305) -> (3:w318:refnum<file>)  [unwired: 4 in, 3 out]
              n106 = Read from Binary File(5:cluster{"x":dbl, "y":dbl, "th":dbl}[] [] ("Points"), 11:w318) -> (3:w304:refnum<file>)  [unwired: 4 in, 3 out]
              n107 = Read from Binary File(5:w317, 11:w304) -> (2:w313:cluster{"Time (s)":dbl, "Distance (ft)":dbl}, 3:w307:refnum<file>)  [unwired: 4 in, 2 out]
              n108 = Unbundle(w313) -> ("Time (s)"=w316:dbl, "Distance (ft)"=w315:dbl)
              n109 = Format Into String(w316) -> (resulting string=w320:string)  [unwired: 3 in, 1 out]
              n110 = Format Into String(w315) -> (resulting string=w319:string)  [unwired: 3 in, 1 out]
            }
          }
          n111 = Close File(refnum=w205) -> ()  [unwired: 1 in, 2 out]
          n112 = Build Array(w200, w202, w201) -> (w209:string[])
        }
        n113 = Replace Array Subset(array=bool[] [FALSE, FALSE, FALSE, FALSE, FALSE, FALSE], new element=TRUE, index="Background") -> (w137:bool[])
        n114 = Index Array(array=w137) -> (element #1=→"IRR":bool, element #2=→"barrels":bool, element #3=→"bounce":bool, element #4=→"slalom":bool, element #5=→"G-S A":bool, element #6=→"G-S B":bool)  [unwired: 6 in]
        n115 = Index Array(array=T19[] [{"Width"=662, "Height"=864}, {"Width"=415, "Height"=835}, {"Width"=415, "Height"=835}, {"Width"=415, "Height"=835}, {"Width"=415, "Height"=835}, {"Width"=415, "Height"=835}], index="Background") -> (element=w131:T19)
        n116 = property on="Picture" class="Pict"("Draw Area Size"=w131) -> ()  [unwired: 2 in, 2 out]
        n117 = property on="Open" class="MCListbox (strict)"("ItemNames"=w180) -> ()  [unwired: 2 in, 2 out]
        n118 = First Call?() -> (First Call?: T/F=w152:bool)
      }
      event "New": Value Change {
        # "Use Initial Location"
        n119 = event-data() -> ()  [unwired: 1 in, 1 out]
        n120 = Unbundle(w326) -> ("Updated Waypoints"=w325:cluster{"x":dbl, "y":dbl, "th":dbl}[])  [unwired: 3 out]
        n121 = local write "Conditions"(T9 {"vInitial (fps)"=0.0, "vFinal (fps)"=0.0} ("Conditions")) -> ()
      }
      event "Append": Value Change {
        n122 = event-data() -> ()  [unwired: 1 in, 1 out]
        n123 = local read "Limits"() -> (w341:T8)
        n124 = Unbundle(w336) -> ("Updated Waypoints"=w335:cluster{"x":dbl, "y":dbl, "th":dbl}[])  [unwired: 3 out]
        n125 = local read "Conditions"() -> (w345:T9)
        n126 = Unbundle(w341) -> ("Velocity (fps)"=w340:dbl, "Accel (fps^2)"=w339:dbl)  [unwired: 2 out]
        n127 = Delete From Array(array=w335) -> (deleted portion=w347:cluster{"x":dbl, "y":dbl, "th":dbl})  [unwired: 2 in, 1 out]
        n128 = Divide(x=w340, y=w339) -> (x/y=w349:dbl)
        n129 = Build Array(w347) -> (w346:cluster{"x":dbl, "y":dbl, "th":dbl}[])
        n130 = Unbundle(w345) -> ("vFinal (fps)"=w344:dbl)  [unwired: 1 out]
        n131 = call "Add First Point.vi"("Accel (f/s^2)"=w339, "Time (s)"=w349, "Initial Points"=w346) -> ("Points"=w348:cluster{"x":dbl, "y":dbl, "th":dbl}[])  [unwired: 8 in]
        n132 = Bundle("vFinal (fps)"=w344, 0.0) -> (w343:cluster{"vFinal (fps)":dbl, dbl})  [unwired: 1 in]
        n133 = local write "Conditions"(w343) -> ()
      }
      event "Play": Value Change {
        n134 = event-data() -> ()  [unwired: 1 in, 1 out]
        n135 = Unbundle(w355) -> ("Updated Waypoints"=w354:cluster{"x":dbl, "y":dbl, "th":dbl}[])  [unwired: 3 out]
        n136 = Tick Count (ms)() -> (millisecond timer value=w356:u32)
        n137 = Generate User Event(user event=w358, event data cluster=w356) -> ()  [unwired: 2 in, 2 out]
      }
      event "Save": Value Change {
        n138 = event-data() -> ()  [unwired: 1 in, 1 out]
        n139 = Unbundle(w392) -> ("Trajectory Data"=w361:T1, "Updated Waypoints"=w390:cluster{"x":dbl, "y":dbl, "th":dbl}[], "Cluster 2"=w362:T30)  [unwired: 1 out]
        n140 = local read "folder names"() -> (w385:cluster{"name":string, "name":string})
        n141 = Unbundle(w385) -> ("name"=w383:string, "name"=w382:string)
        n142 = call "Append String To Path.vi"("name"=w383, "path in"=w384) -> ("appended path out"=w381:path)  [unwired: 9 in]
        n143 = Unbundle(w362) -> ("Sample Period (s)"=w366:dbl, "Limits"=w365:T8, "Conditions"=w364:T9, "Overrides"=w370:T7)
        n144 = call "Append String To Path.vi"("name"=w382, "path in"=w381) -> ("appended path out"=w380:path)  [unwired: 9 in]
        n145 = for {
          tunnel: w370 -> [w400] mode=indexing
          tunnel: [w399] -> w369 mode=indexing
          tunnel: [w398] -> w368 mode=indexing
          n146 = Unbundle(w400) -> ("Angular Multiplier"=w399:dbl, "1"=w398:bool)  [unwired: 2 out]
        }
        n147 = Bundle("Robot Backwards"="Robot Backwards", "Reverse Path"="Reverse Path") -> (w371:T32)  [unwired: 1 in]
        n148 = Build Path(base path=w380, name or relative path="Filename") -> (appended path=w395:path)
        n149 = Bundle(w369, w368) -> (w367:cluster{dbl[], bool[]})  [unwired: 1 in]
        n150 = Write to Binary File(file (use dialog)=w395, data="3.2") -> (refnum out=w379:refnum<file>)  [unwired: 4 in, 2 out]
        n151 = Bundle("Sample Period (s)"=w366, "Limits"=w365, "Conditions"=w364, w367) -> (w363:T33)  [unwired: 1 in]
        n152 = Write to Binary File(file (use dialog)=w379, data=w371) -> (refnum out=w376:refnum<file>)  [unwired: 4 in, 2 out]
        n153 = Write to Binary File(file (use dialog)=w376, data=w361) -> (refnum out=w375:refnum<file>)  [unwired: 4 in, 2 out]
        n154 = Write to Binary File(file (use dialog)=w375, data=w360) -> (refnum out=w374:refnum<file>)  [unwired: 4 in, 2 out]
        n155 = Write to Binary File(file (use dialog)=w374, data=w363) -> (refnum out=w396:refnum<file>)  [unwired: 4 in, 2 out]
        n156 = Write to Binary File(file (use dialog)=w396, data=w390) -> (refnum out=w378:refnum<file>)  [unwired: 4 in, 2 out]
        n157 = Bundle("Trajectory Data"=w361, "Updated Waypoints"=w390, "Cluster 2"=w362, w360) -> (w393:T34)  [unwired: 1 in]
        n158 = Write to Binary File(file (use dialog)=w378, data=w386) -> (refnum out=w377:refnum<file>)  [unwired: 4 in, 2 out]
        n159 = Close File(refnum=w377) -> ()  [unwired: 1 in, 2 out]
      }
      event "Open Command": Value Change {
        n160 = event-data() -> ()  [unwired: 1 in, 1 out]
        n161 = Unbundle(w410) -> ("Updated Waypoints"=w409:cluster{"x":dbl, "y":dbl, "th":dbl}[])  [unwired: 3 out]
        n162 = call "Open Command Panel.vi"("Commands"=w408, "Tag"="Command Sequence") -> ("Found"=w405:bool)  [unwired: 9 in]
        n163 = Select(t="Command Sequence", s=w405, f="") -> (s? t:f=w402:string)
        n164 = Bundle(cluster=w406, "Filename"=w402) -> (w407:T15)  [unwired: 2 in]
      }
      event "Directory": Value Change {
        n165 = event-data() -> ()  [unwired: 1 in, 1 out]
        n166 = Unbundle(w427) -> ("Updated Waypoints"=w426:cluster{"x":dbl, "y":dbl, "th":dbl}[])  [unwired: 3 out]
        n167 = call "File Dialog"("start path"=w420, "prompt"="Path Folder", "button label"="Select") -> ("selected path"=w419:path, "error out"=w421:errorcluster)  [unwired: 9 in, 2 out]
        n168 = Select(t=w420, s=w421, f=w419) -> (s? t:f=w418:path)
        n169 = Format Into String(format string=w423, w418) -> (resulting string=w424:string)  [unwired: 2 in, 1 out]
        n170 = property class="VI"("Front Panel.Title"=w424) -> ()  [unwired: 2 in, 2 out]
      }
      event "Open": Double Click {
        # "Need the Waypoints in the file TODO"
        n171 = event-data() -> ("Row"=w467:i32)  [unwired: 1 in]
        n172 = property on="Open" class="MCListbox (strict)"() -> ("ItemNames"=w468:string[][])  [unwired: 2 in, 2 out]
        n173 = local read "folder names"() -> (w449:cluster{"name":string, "name":string})
        n174 = Index Array(array=w468, index (row)=w467, index (col)=0 ("disabled index (col)")) -> (element=w458:string)
        n175 = Unbundle(w449) -> ("name"=w439:string, "name"=w442:string)
        n176 = call "Append String To Path.vi"("name"=w439, "path in"=w441) -> ("appended path out"=w440:path)  [unwired: 9 in]
        n177 = call "Append String To Path.vi"("name"=w442, "path in"=w440) -> ("appended path out"=w448:path)  [unwired: 9 in]
        n178 = Build Path(base path=w448, name or relative path=w458) -> (appended path=w459:path)
        n179 = local write "Filename"(w458) -> ()
        n180 = Unbundle(w452) -> ("Trajectory Data"=w445:T1, "Cluster 2"=w451:T30)  [unwired: 2 out]
        n181 = Read from Binary File(5:"", 11:w459) -> (2:w464:string, 3:w463:refnum<file>)  [unwired: 4 in, 2 out]
        n182 = case shown="\"3.2\"" w464 {
          tunnel: w463 -> [w471 w488 w508 w528 w549 w576 w600 w625 w651 w670 w699]
          tunnel: w451 -> [_ _ _ _ _ _ _ _ _ _ _]
          tunnel: w462 -> [_ w486 w506 w526 w547 w574 w598 w623 w649 w679 w708]
          tunnel: [_ w485 w505 w525 w546 w573 w597 w622 w648 w678 w707] -> w453
          tunnel: w445 -> [_ w484 w504 w524 w545 w572 w596 w621 w647 w677 w706]
          tunnel: w460 -> [_ w482 w502 w522 w543 w570 w594 w619 w645 w676 w705]
          tunnel: [w471 w480 w500 w520 w541 w568 w588 w613 w639 w666 w695] -> w461
          tunnel: [_ w478 w499 w519 w540 w567 w592 w617 w643 w653 w682] -> w457
          tunnel: [_ w474 w493 w512 w534 w562 w582 w608 w627 w658 w687] -> w438
          tunnel: [_ _ w498 w518 w539 w566 w591 w616 w642 w675 w704] -> w456
          tunnel: [w469 w473 w492 w511 w533 w560 w579 w605 w633 w662 w691] -> w432
          tunnel: [T1 [] ("Trajectory Data") w476 w496 w516 w537 w565 w590 w615 w641 w674 w703] -> w454
          tunnel: [_ _ _ _ _ _ w587 _ _ _ _] -> _
          tunnel: w444 -> [_ _ _ _ _ _ _ w612 w638 w673 w702]
          tunnel: [_ _ _ _ _ _ _ w611 w637 w672 w701] -> w437
          tunnel: [_ _ _ _ _ _ _ w610 w636 w671 w700] -> _
          tunnel: T23 {"Sample Period (s)"=0.0, "Limits 2"={"Velocity (fps)"=0.0, "Acceleration (fps^2)"=0.0, "Jerk (fps^3)"=0.0}, "Conditions"={"vInitial (fps)"=0.0, "vFinal (fps)"=0.0}, " Acceleration Overrides"={"Angular \nAccelerations"=[], "Accel Override Bools"=[]}} ("Cluster") -> [_ _ _ _ _ w564 w585 w606 _ _ _]
          tunnel: [_ _ _ _ _ _ _ _ _ w661 w690] -> w435
          tunnel: T7 [] ("Overrides") -> [w469 w473 w492 w511 _ _ _ _ _ _ _]
          frame "False", Default {
          }
          frame "2.0", "2.1" {
            n183 = Read from Binary File(5:T20 {"Velocity"=0.0, "Sample Time"=0.0, "Accel"=0.0}, 11:w488) -> (2:w489:T20, 3:w487:refnum<file>)  [unwired: 4 in, 2 out]
            n184 = Read from Binary File(5:w486, 11:w487) -> (2:w485:cluster{"x":dbl, "y":dbl, "th":dbl}[], 3:w483:refnum<file>)  [unwired: 4 in, 2 out]
            n185 = Unbundle(w489) -> ("Velocity"=w475:dbl, "Sample Time"=w478:dbl, "Accel"=w472:dbl)
            n186 = Read from Binary File(5:w484, 11:w483) -> (2:w476:T1, 3:w481:refnum<file>)  [unwired: 4 in, 2 out]
            n187 = Read from Binary File(5:w482, 11:w481) -> (3:w480:refnum<file>)  [unwired: 4 in, 3 out]
            n188 = Bundle("Velocity"=w475, "Accel"=w472, "Accel"=1000.0, "Velocity"=w475) -> (w474:T35)  [unwired: 1 in]
          }
          frame "2.3" {
            n189 = Read from Binary File(5:T21 {"Sample Period (s)"=0.0, "Limits"={"Velocity (fps)"=0.0, "Acceleration (fps^2)"=0.0, "Jerk (fps^3)"=0.0}, "Conditions"={"vInitial (fps)"=0.0, "vFinal (fps)"=0.0}}, 11:w508) -> (2:w509:T21, 3:w507:refnum<file>)  [unwired: 4 in, 2 out]
            n190 = Unbundle(w509) -> ("Sample Period (s)"=w499:dbl, "Limits"=w490:T36, "Conditions"=w498:T9)
            n191 = Read from Binary File(5:w506, 11:w507) -> (2:w505:cluster{"x":dbl, "y":dbl, "th":dbl}[], 3:w503:refnum<file>)  [unwired: 4 in, 2 out]
            n192 = Read from Binary File(5:w504, 11:w503) -> (2:w496:T1, 3:w501:refnum<file>)  [unwired: 4 in, 2 out]
            n193 = Read from Binary File(5:w502, 11:w501) -> (3:w500:refnum<file>)  [unwired: 4 in, 3 out]
            n194 = Unbundle(w490) -> ("Velocity (fps)"=w495:dbl, "Acceleration (fps^2)"=w491:dbl, "Jerk (fps^3)"=w494:dbl)
            n195 = Bundle("Velocity (fps)"=w495, "Acceleration (fps^2)"=w491, "Jerk (fps^3)"=w494, "Velocity (fps)"=w495) -> (w493:T37)  [unwired: 1 in]
          }
          frame "2.4" {
            n196 = Read from Binary File(5:T21 {"Sample Period (s)"=0.0, "Limits"={"Velocity (fps)"=0.0, "Acceleration (fps^2)"=0.0, "Jerk (fps^3)"=0.0}, "Conditions"={"vInitial (fps)"=0.0, "vFinal (fps)"=0.0}}, 11:w528) -> (2:w529:T21, 3:w527:refnum<file>)  [unwired: 4 in, 2 out]
            n197 = Unbundle(w529) -> ("Sample Period (s)"=w519:dbl, "Limits"=w513:T36, "Conditions"=w518:T9)
            n198 = Read from Binary File(5:w526, 11:w527) -> (2:w525:cluster{"x":dbl, "y":dbl, "th":dbl}[], 3:w523:refnum<file>)  [unwired: 4 in, 2 out]
            n199 = Read from Binary File(5:w524, 11:w523) -> (2:w516:T1, 3:w521:refnum<file>)  [unwired: 4 in, 2 out]
            n200 = Read from Binary File(5:w522, 11:w521) -> (3:w520:refnum<file>)  [unwired: 4 in, 3 out]
            n201 = Unbundle(w513) -> ("Velocity (fps)"=w515:dbl, "Acceleration (fps^2)"=w510:dbl, "Jerk (fps^3)"=w514:dbl)
            n202 = Bundle("Velocity (fps)"=w515, "Acceleration (fps^2)"=w510, "Jerk (fps^3)"=w514, "Velocity (fps)"=w515) -> (w512:T37)  [unwired: 1 in]
          }
          frame "2.5" {
            n203 = Read from Binary File(5:T24 {"Sample Period (s)"=0.0, "Limits"={"Velocity (fps)"=0.0, "Acceleration (fps^2)"=0.0, "Jerk (fps^3)"=0.0}, "Conditions"={"vInitial (fps)"=0.0, "vFinal (fps)"=0.0}, "Min Rads"=[20.0, 20.0, 20.0, 20.0, 20.0]}, 11:w549) -> (2:w550:T24, 3:w548:refnum<file>)  [unwired: 4 in, 2 out]
            n204 = Unbundle(w550) -> ("Sample Period (s)"=w540:dbl, "Limits"=w535:T36, "Conditions"=w539:T9, "Min Rads"=w532:dbl[])
            n205 = Read from Binary File(5:w547, 11:w548) -> (2:w546:cluster{"x":dbl, "y":dbl, "th":dbl}[], 3:w544:refnum<file>)  [unwired: 4 in, 2 out]
            n206 = Read from Binary File(5:w545, 11:w544) -> (2:w537:T1, 3:w542:refnum<file>)  [unwired: 4 in, 2 out]
            n207 = Unbundle(w535) -> ("Velocity (fps)"=w531:dbl, "Acceleration (fps^2)"=w530:dbl, "Jerk (fps^3)"=w536:dbl)
            n208 = for {
              tunnel: [w555] -> w533 mode=indexing
              tunnel: w532 -> [w554] mode=indexing
              tunnel: w531 -> [w553]
              i -> [w552]
              n209 = Format Into String(w552) -> (resulting string=w551:string)  [unwired: 3 in, 1 out]
              n210 = Bundle(w551, "Angular Multiplier"=w554, TRUE, "Velocity (fps)"=w553) -> (w555:T38)  [unwired: 1 in]
            }
            n211 = Read from Binary File(5:w543, 11:w542) -> (3:w541:refnum<file>)  [unwired: 4 in, 3 out]
            n212 = Bundle("Velocity (fps)"=w531, "Acceleration (fps^2)"=w530, "Jerk (fps^3)"=w536, "Velocity (fps)"=w531) -> (w534:T37)  [unwired: 1 in]
          }
          frame "2.6" {
            n213 = Read from Binary File(5:w564, 11:w576) -> (2:w577:T23, 3:w575:refnum<file>)  [unwired: 4 in, 2 out]
            n214 = Unbundle(w577) -> ("Sample Period (s)"=w567:dbl, "Limits 2"=w561:T36, "Conditions"=w566:T9, "Acceleration Overrides"=w558:T39)
            n215 = Read from Binary File(5:w574, 11:w575) -> (2:w573:cluster{"x":dbl, "y":dbl, "th":dbl}[], 3:w571:refnum<file>)  [unwired: 4 in, 2 out]
            n216 = Read from Binary File(5:w572, 11:w571) -> (2:w565:T1, 3:w569:refnum<file>)  [unwired: 4 in, 2 out]
            n217 = Read from Binary File(5:w570, 11:w569) -> (3:w568:refnum<file>)  [unwired: 4 in, 3 out]
            n218 = Unbundle(w561) -> ("Velocity (fps)"=w559:dbl, "Acceleration (fps^2)"=w557:dbl, "Jerk (fps^3)"=w563:dbl)
            n219 = Bundle("Velocity (fps)"=w559, "Acceleration (fps^2)"=w557, "Jerk (fps^3)"=w563, "Velocity (fps)"=w559) -> (w562:T37)  [unwired: 1 in]
            n220 = call "Convert Overrides.vi"("Cluster"=w558, "Velocity (fps)"=w559) -> ("Array"=w560:T40)  [unwired: 9 in]
          }
          frame "2.7" {
            n221 = Read from Binary File(5:w585, 11:w600) -> (2:w601:T23, 3:w599:refnum<file>)  [unwired: 4 in, 2 out]
            n222 = Unbundle(w601) -> ("Sample Period (s)"=w592:dbl, "Limits 2"=w583:T36, "Conditions"=w591:T9, "Acceleration Overrides"=w580:T39)
            n223 = Read from Binary File(5:w598, 11:w599) -> (2:w597:cluster{"x":dbl, "y":dbl, "th":dbl}[], 3:w595:refnum<file>)  [unwired: 4 in, 2 out]
            n224 = Read from Binary File(5:w596, 11:w595) -> (2:w590:T1, 3:w593:refnum<file>)  [unwired: 4 in, 2 out]
            n225 = Read from Binary File(5:w594, 11:w593) -> (3:w589:refnum<file>)  [unwired: 4 in, 3 out]
            n226 = Unbundle(w583) -> ("Velocity (fps)"=w581:dbl, "Acceleration (fps^2)"=w578:dbl, "Jerk (fps^3)"=w584:dbl)
            n227 = Read from Binary File(5:T26 [] ("Commands"), 11:w589) -> (2:w587:T26, 3:w588:refnum<file>)  [unwired: 4 in, 2 out]
            n228 = Bundle("Velocity (fps)"=w581, "Acceleration (fps^2)"=w578, "Jerk (fps^3)"=w584, "Velocity (fps)"=w581) -> (w582:T37)  [unwired: 1 in]
            n229 = call "Convert Overrides.vi"("Cluster"=w580, "Velocity (fps)"=w581) -> ("Array"=w579:T40)  [unwired: 9 in]
          }
          frame "2.8" {
            n230 = Read from Binary File(5:w606, 11:w625) -> (2:w626:T23, 3:w624:refnum<file>)  [unwired: 4 in, 2 out]
            n231 = Unbundle(w626) -> ("Sample Period (s)"=w617:dbl, "Limits 2"=w609:T36, "Conditions"=w616:T9, "Acceleration Overrides"=w603:T39)
            n232 = Read from Binary File(5:w623, 11:w624) -> (2:w622:cluster{"x":dbl, "y":dbl, "th":dbl}[], 3:w620:refnum<file>)  [unwired: 4 in, 2 out]
            n233 = Read from Binary File(5:w621, 11:w620) -> (2:w615:T1, 3:w618:refnum<file>)  [unwired: 4 in, 2 out]
            n234 = Read from Binary File(5:w619, 11:w618) -> (3:w614:refnum<file>)  [unwired: 4 in, 3 out]
            n235 = Unbundle(w609) -> ("Velocity (fps)"=w604:dbl, "Acceleration (fps^2)"=w602:dbl, "Jerk (fps^3)"=w607:dbl)
            n236 = Read from Binary File(5:w612, 11:w614) -> (0:w610:errorcluster, 2:w611:cluster{"Time (s)":dbl, T3, bool}[], 3:w613:refnum<file>)  [unwired: 4 in, 1 out]
            n237 = call "Convert Overrides.vi"("Cluster"=w603, "Velocity (fps)"=w604) -> ("Array"=w605:T40)  [unwired: 9 in]
            n238 = Bundle("Velocity (fps)"=w604, "Acceleration (fps^2)"=w602, "Jerk (fps^3)"=w607, "Velocity (fps)"=w604) -> (w608:T37)  [unwired: 1 in]
          }
          frame "3.0" {
            n239 = Read from Binary File(5:T27 {"Sample Period (s)"=0.0, "Limits 2"={"Velocity (fps)"=0.0, "Acceleration (fps^2)"=0.0, "Jerk (fps^3)"=0.0, "Stoopid Fast"=0.0}, "Conditions"={"vInitial (fps)"=0.0, "vFinal (fps)"=0.0}, " Acceleration Overrides"={"Angular \nAccelerations"=[], "Accel Override Bools"=[]}} ("Cluster"), 11:w651) -> (2:w652:T27, 3:w650:refnum<file>)  [unwired: 4 in, 2 out]
            n240 = Unbundle(w652) -> ("Sample Period (s)"=w643:dbl, "Limits 2"=w628:T41, "Conditions"=w642:T9, "Acceleration Overrides"=w634:T39)
            n241 = Read from Binary File(5:w649, 11:w650) -> (2:w648:cluster{"x":dbl, "y":dbl, "th":dbl}[], 3:w646:refnum<file>)  [unwired: 4 in, 2 out]
            n242 = Read from Binary File(5:w647, 11:w646) -> (2:w641:T1, 3:w644:refnum<file>)  [unwired: 4 in, 2 out]
            n243 = Read from Binary File(5:w645, 11:w644) -> (3:w640:refnum<file>)  [unwired: 4 in, 3 out]
            n244 = Unbundle(w628) -> ("Velocity (fps)"=w632:dbl, "Acceleration (fps^2)"=w631:dbl, "Jerk (fps^3)"=w630:dbl, "Stoopid Fast"=w629:dbl)
            n245 = call "Convert Overrides.vi"("Cluster"=w634, "Velocity (fps)"=w632) -> ("Array"=w633:T40)  [unwired: 9 in]
            n246 = Read from Binary File(5:w638, 11:w640) -> (0:w636:errorcluster, 2:w637:cluster{"Time (s)":dbl, T3, bool}[], 3:w639:refnum<file>)  [unwired: 4 in, 1 out]
            n247 = Bundle("Velocity (fps)"=w632, "Acceleration (fps^2)"=w631, "Jerk (fps^3)"=w630, "Stoopid Fast"=w629) -> (w627:T41)  [unwired: 1 in]
          }
          frame "3.1" {
            n248 = Read from Binary File(5:T22 {"Reverse Path"=FALSE, "Robot Backwards"=FALSE} ("Cluster"), 11:w670) -> (2:w661:T22, 3:w667:refnum<file>)  [unwired: 4 in, 2 out]
            n249 = Read from Binary File(5:w677, 11:w667) -> (2:w674:T1, 3:w665:refnum<file>)  [unwired: 4 in, 2 out]
            n250 = Read from Binary File(5:w673, 11:w665) -> (0:w671:errorcluster, 2:w672:cluster{"Time (s)":dbl, T3, bool}[], 3:w664:refnum<file>)  [unwired: 4 in, 1 out]
            n251 = Read from Binary File(5:T17 {"Sample Period (s)"=0.0, "Limits"={"Velocity (fps)"=0.0, "Accel (fps^2)"=0.0, "Turn Accel (fps^2)"=15.0, "Jerk (fps^3)"=0.0}, "Conditions"={"vInitial (fps)"=0.0, "vFinal (fps)"=0.0}, {[], []}} ("Cluster 2"), 11:w664) -> (2:w681:T17, 3:w680:refnum<file>)  [unwired: 4 in, 2 out]
            n252 = Unbundle(w681) -> ("Sample Period (s)"=w653:dbl, "Limits"=w660:T42, "Conditions"=w675:T9, w663:cluster{dbl[], bool[]})
            n253 = Read from Binary File(5:w679, 11:w680) -> (2:w678:cluster{"x":dbl, "y":dbl, "th":dbl}[], 3:w668:refnum<file>)  [unwired: 4 in, 2 out]
            n254 = Read from Binary File(5:w676, 11:w668) -> (3:w666:refnum<file>)  [unwired: 4 in, 3 out]
            n255 = Unbundle(w660) -> ("Velocity (fps)"=w657:dbl, "Accel (fps^2)"=w656:dbl, "Turn Accel (fps^2)"=w655:dbl, "Jerk (fps^3)"=w654:dbl)
            n256 = call "Convert Overrides.vi"("Cluster"=w663, "Velocity (fps)"=w657) -> ("Array"=w662:T40)  [unwired: 9 in]
            n257 = Bundle("Velocity (fps)"=w657, "Accel (fps^2)"=w656, "Turn Accel (fps^2)"=w655, "Jerk (fps^3)"=w654) -> (w658:T42)  [unwired: 1 in]
          }
          frame "3.2" {
            n258 = Read from Binary File(5:T22 {"Reverse Path"=FALSE, "Robot Backwards"=FALSE} ("Cluster"), 11:w699) -> (2:w690:T22, 3:w696:refnum<file>)  [unwired: 4 in, 2 out]
            n259 = Read from Binary File(5:w706, 11:w696) -> (2:w703:T1, 3:w694:refnum<file>)  [unwired: 4 in, 2 out]
            n260 = Read from Binary File(5:w702, 11:w694) -> (0:w700:errorcluster, 2:w701:cluster{"Time (s)":dbl, T3, bool}[], 3:w693:refnum<file>)  [unwired: 4 in, 1 out]
            n261 = Read from Binary File(5:T17 {"Sample Period (s)"=0.0, "Limits"={"Velocity (fps)"=0.0, "Accel (fps^2)"=0.0, "Turn Accel (fps^2)"=15.0, "Jerk (fps^3)"=0.0}, "Conditions"={"vInitial (fps)"=0.0, "vFinal (fps)"=0.0}, {[], []}} ("Cluster 2"), 11:w693) -> (2:w710:T17, 3:w709:refnum<file>)  [unwired: 4 in, 2 out]
            n262 = Unbundle(w710) -> ("Sample Period (s)"=w682:dbl, "Limits"=w689:T42, "Conditions"=w704:T9, w692:cluster{dbl[], bool[]})
            n263 = Read from Binary File(5:w708, 11:w709) -> (2:w707:cluster{"x":dbl, "y":dbl, "th":dbl}[], 3:w697:refnum<file>)  [unwired: 4 in, 2 out]
            n264 = Read from Binary File(5:w705, 11:w697) -> (3:w695:refnum<file>)  [unwired: 4 in, 3 out]
            n265 = Unbundle(w689) -> ("Velocity (fps)"=w686:dbl, "Accel (fps^2)"=w685:dbl, "Turn Accel (fps^2)"=w684:dbl, "Jerk (fps^3)"=w683:dbl)
            n266 = call "Convert Overrides.vi"("Cluster"=w692, "Velocity (fps)"=w686) -> ("Array"=w691:T40)  [unwired: 9 in]
            n267 = Bundle("Velocity (fps)"=w686, "Accel (fps^2)"=w685, "Turn Accel (fps^2)"=w684, "Jerk (fps^3)"=w683) -> (w687:T42)  [unwired: 1 in]
          }
        }
        n268 = Close File(refnum=w461) -> ()  [unwired: 1 in, 2 out]
        n269 = Bundle("Sample Period (s)"=w457, w438, "Conditions"=w456, "Array"=w432) -> (w455:T43)  [unwired: 1 in]
        n270 = Unbundle(w435) -> ("Reverse Path"=w434:bool, "Robot Backwards"=w433:bool)
        n271 = local write "Robot Backwards"(w434) -> ()
        n272 = local write "Sample Period (s)"(w457) -> ()
        n273 = local write "Limits"(w438) -> ()
        n274 = local write "Conditions"(w456) -> ()
        n275 = local write "Reverse Path"(w433) -> ()
        n276 = local write "Overrides"(w432) -> ()
        n277 = Bundle("Trajectory Data"=w454, "Points"=w453, w455, w437) -> (w430:T44)  [unwired: 1 in]
      }
      event "Picture": Mouse Down {
        n278 = event-data() -> ("Coords"=w725:T45, "Button"=w727:u16, "Mods"=w726:cluster{"Double Click":bool, "Menu Key":bool}, "PlatMods"=w722:T46)  [unwired: 1 in]
        n279 = Unbundle(w719) -> ("Updated Waypoints"=w718:cluster{"x":dbl, "y":dbl, "th":dbl}[])  [unwired: 3 out]
        n280 = Unbundle(w715) -> ("Drag Object"=w714:cluster{"Index":i32, "x":dbl, "y":dbl})  [unwired: 2 out]
        n281 = case shown="1" w727 {
          tunnel: w726 -> [_ _ w739]
          tunnel: w725 -> [_ _ w744]
          tunnel: w718 -> [w731 w735 w745]
          tunnel: [w731 w735 w749] -> w724
          tunnel: w723 -> [_ _ w746]
          tunnel: w714 -> [w729 w732 w740]
          tunnel: [w728 w734 w741] -> w716
          tunnel: w722 -> [_ _ w737]
          frame 0, Default {
            # "middle mouse?"
            n282 = Bundle(cluster=w729, "Index"=-1) -> (w728:cluster{"Index":i32, "x":dbl, "y":dbl})  [unwired: 2 in]
          }
          frame 2 {
            # "Right Button"
            n283 = Bundle(cluster=w732, "Index"=-1) -> (w734:cluster{"Index":i32, "x":dbl, "y":dbl})  [unwired: 2 in]
          }
          frame 1 {
            # "Left Button"
            n284 = Unbundle By Name(w739) -> ("Double Click"=w738:bool)
            n285 = property on="Picture" class="Pict"() -> ("Position"=w748:T12, "Draw Area Size"=w747:T19)  [unwired: 2 in, 2 out]
            n286 = Unbundle By Name(w737) -> ("Shift"=w736:bool)
            n287 = call "Point Test Shapes.vi"("Coords"=w744, "Points"=w745, "Picture in"=w746) -> ("Pt Test Results"=w743:enum16{"Miss", "Rect Hit", "Arrow Hit"}, "Results"=w742:T14)  [unwired: 7 in]
            n288 = case shown="\"Miss\", Default" w743 {
              tunnel: w738 -> [_ _ w792]
              tunnel: w745 -> [w753 w781 w786]
              tunnel: w742 -> [_ w779 w793]
              tunnel: [w756 w782 w785] -> w749
              tunnel: w744 -> [w757 _ _]
              tunnel: w748 -> [w755 _ _]
              tunnel: w747 -> [w754 _ _]
              tunnel: [w751 w774 w789] -> w741
              tunnel: w740 -> [w750 _ w790]
              tunnel: w736 -> [w752 _ w787]
              frame "Miss", Default {
                n289 = case shown="True" w752 {
                  tunnel: w757 -> [w769 _]
                  tunnel: [w766 w773] -> w756
                  tunnel: w755 -> [w765 _]
                  tunnel: w754 -> [w764 _]
                  tunnel: w753 -> [w760 w773]
                  tunnel: [w759 w772] -> w751
                  tunnel: w750 -> [_ w770]
                  frame False {
                    n290 = call "Map to Feet.vi"("Draw Area Size"=w764, "Position"=w765, "Coords (px)"=w769) -> ("Point (ft)"=w763:cluster{dbl, dbl})  [unwired: 8 in]
                    n291 = Array Size(array=w760) -> (size(s)=w758:i32)
                    n292 = Unbundle(w763) -> (w762:dbl, w761:dbl)
                    n293 = Bundle(w762, w761, nan) -> (w767:cluster{dbl, dbl, dbl})  [unwired: 1 in]
                    n294 = Bundle(w758, w762, w761) -> (w759:cluster{i32, dbl, dbl})  [unwired: 1 in]
                    n295 = Build Array (concatenate)(w760, w767) -> (w766:cluster{"x":dbl, "y":dbl, "th":dbl}[])
                  }
                  frame True {
                    n296 = Bundle(cluster=w770, "Index"=-1) -> (w772:cluster{"Index":i32, "x":dbl, "y":dbl})  [unwired: 2 in]
                  }
                }
              }
              frame "Arrow Hit" {
                # "start tracking rotation"
                n297 = Unbundle(w779) -> ("Index"=w778:i32)  [unwired: 1 out]
                n298 = Index Array(array=w781, index=w778) -> (element=w780:cluster{"x":dbl, "y":dbl, "th":dbl})
                n299 = Unbundle(w780) -> ("x"=w777:dbl, "y"=w776:dbl, "th"=w784:dbl)
                n300 = Bundle(cluster=w780, "th"=w784) -> (w783:cluster{"x":dbl, "y":dbl, "th":dbl})  [unwired: 2 in]
                n301 = Bundle(-2, "x"=w777, "y"=w776) -> (w774:cluster{i32, "x":dbl, "y":dbl})  [unwired: 1 in]
                n302 = Replace Array Subset(array=w781, new element=w783) -> (w782:cluster{"x":dbl, "y":dbl, "th":dbl}[])  [unwired: 1 in]
              }
              frame "Rect Hit" {
                n303 = Unbundle(w793) -> ("Index"=w791:i32)  [unwired: 1 out]
                n304 = case shown="False" w787 {
                  tunnel: w792 -> [w797 _]
                  tunnel: w791 -> [w796 w800]
                  tunnel: [w795 -1 ("length")] -> w788
                  tunnel: w786 -> [w794 w803]
                  tunnel: [w794 w802] -> w785
                  frame False {
                    n305 = case shown="False" w797 {
                      tunnel: w796 -> [w798 _]
                      tunnel: [w798 -1] -> w795
                      frame False {
                      }
                      frame True {
                        # "TODO Toggle last pt"
                      }
                    }
                  }
                  frame True {
                    n306 = case shown="Default" w800 {
                      tunnel: w803 -> [w804 w808]
                      tunnel: w800 -> [_ w807]
                      tunnel: [w804 w805] -> w802
                      frame 0 {
                      }
                      frame Default {
                        n307 = Delete From Array(array=w808, length=1, index=w807) -> (array with subset deleted=w805:cluster{"x":dbl, "y":dbl, "th":dbl}[])  [unwired: 1 out]
                      }
                    }
                  }
                }
                n308 = Bundle(cluster=w790, "Index"=w788) -> (w789:cluster{"Index":i32, "x":dbl, "y":dbl})  [unwired: 2 in]
              }
            }
          }
        }
        n309 = Bundle(cluster=w715, "Drag Object"=w716) -> (w717:T15)  [unwired: 2 in]
      }
      event "Picture": Mouse Move; "Picture": Mouse Up {
        n310 = event-data() -> ("Type"=w826:T28, "Coords"=w828:T45)  [unwired: 1 in]
        n311 = Unbundle(w819) -> ("Updated Waypoints"=w818:cluster{"x":dbl, "y":dbl, "th":dbl}[])  [unwired: 3 out]
        n312 = Unbundle(w811) -> ("Drag Object"=w814:cluster{"Index":i32, "x":dbl, "y":dbl})  [unwired: 2 out]
        n313 = Unbundle(w814) -> ("Index"=w825:i32)  [unwired: 2 out]
        n314 = case shown="Default" w825 {
          selector: w825 -> [w838 _]
          tunnel: w828 -> [w847 w855]
          tunnel: [w845 w854] -> w816
          tunnel: [w842 w853] -> w827
          tunnel: w818 -> [w843 w853]
          tunnel: [w839 w852] -> w817
          tunnel: w814 -> [w830 w852]
          tunnel: w826 -> [w840 _]
          tunnel: "Snap to foot" -> [w835 _]
          tunnel: "Snap robot to baseline" -> [w836 _]
          tunnel: "Angle Limiter" -> [w837 _]
          tunnel: w810 -> [w829 w851]
          tunnel: w809 -> [_ w850]
          frame Default {
            # "Mouse up changes indes to break tracking,\notherwise update coords"
            n315 = property on="Picture" class="Pict"() -> ("Position"=w848:T12, "Draw Area Size"=w849:T19)  [unwired: 2 in, 2 out]
            n316 = Bundle("Snap robot to baseline"=w836, "Snap to foot"=w835, "Angle Limiter"=w837) -> (w834:T47)  [unwired: 1 in]
            n317 = call "Map to Feet.vi"("Draw Area Size"=w849, "Position"=w848, "Coords (px)"=w847) -> ("Point (ft)"=w846:cluster{dbl, dbl})  [unwired: 8 in]
            n318 = Equal?(x=lveventtype."Mouse Up" ("Type"), y=w840) -> (x = y?=w833:bool)
            n319 = call "Handle Pos and Rot.vi"("Mouse Up"=w833, "Picture in"=w829, "Option"=w834, "Coord (ft)"=w846, "Index"=w838, "Points in"=w843) -> ("Points out"=w842:cluster{"x":dbl, "y":dbl, "th":dbl}[])  [unwired: 5 in]
            n320 = Bundle(cluster=w830, "Index"=-1) -> (w831:cluster{"Index":i32, "x":dbl, "y":dbl})  [unwired: 2 in]
            n321 = Bundle(w838, "Pt Test Results"=enum16{"Miss", "Rect Hit", "Arrow Hit"}."Rect Hit") -> (w845:T48)  [unwired: 1 in]
            n322 = Select(t=w831, s=w833, f=w830) -> (s? t:f=w839:cluster{"Index":i32, "x":dbl, "y":dbl})
          }
          frame -1 {
            n323 = call "Point Test Shapes.vi"("Array"=w850, "Coords"=w855, "Points"=w853, "Picture in"=w851) -> ("Results"=w854:T14)  [unwired: 6 in, 1 out]
          }
        }
        n324 = Bundle(cluster=w811, "Drag Object"=w817, "Hover Object"=w816) -> (w815:T15)  [unwired: 1 in]
      }
      event "Time (s)", "Snap to foot", "Angle Limiter", "Snap robot to baseline", "Sample Period (s)", "Center Flip", "Conditions", "Unjank", "Allow Angles > 90", "Overrides": Value Change {
        # "Changes to any of these control will run the diagram to update the preview"
        n325 = event-data() -> ("CtlRef"=w869:refnum<vi>)  [unwired: 1 in]
        n326 = control-ref of="Center Flip"() -> (w870:refnum<vi>)
        n327 = Equal?(x=w870, y=w869) -> (x = y?=w868:bool)
        n328 = Unbundle(w863) -> ("Updated Waypoints"=w862:cluster{"x":dbl, "y":dbl, "th":dbl}[])  [unwired: 3 out]
        n329 = case shown="True" "Unjank" {
          tunnel: w863 -> [_ w875]
          tunnel: "Turn Acceleration" -> [_ w874]
          tunnel: "Turn Deceleration" -> [_ w873]
          frame False {
          }
          frame True {
            n330 = call "Turn Smother.vi"("Ignore Deceleration"=w873, "Ignore Acceleration"=w874, "input cluster"=w875) -> ("Overrides"=w872:T7)  [unwired: 1 in]
            n331 = local write "Overrides"(w872) -> ()
          }
        }
        n332 = case shown="True" w868 {
          tunnel: w862 -> [w876 w878]
          tunnel: [w876 w877] -> w871
          frame False {
          }
          frame True {
            n333 = for {
              tunnel: w878 -> [w886] mode=indexing
              tunnel: [w879] -> w877 mode=indexing
              n334 = Unbundle(w886) -> ("x"=w885:dbl, "y"=w881:dbl, "th"=w880:dbl)
              n335 = Negate(x=w885) -> (-x=w884:dbl)
              n336 = Add(x=27.0 ("y"), y=w884) -> (x+y=w882:dbl)
              n337 = Bundle(w882, "y"=w881, "th"=w880) -> (w879:cluster{dbl, "y":dbl, "th":dbl})  [unwired: 1 in]
            }
          }
        }
      }
      event Key Down?; event type 5.0.x8000000b {
        n338 = event-data() -> ("VKey"=w900:T49)  [unwired: 1 in]
        n339 = local read "Snap robot to baseline"() -> (w907:bool)
        n340 = Unbundle(w894) -> ("Updated Waypoints"=w893:cluster{"x":dbl, "y":dbl, "th":dbl}[])  [unwired: 3 out]
        n341 = local read "Angle Limiter"() -> (w905:enum16{"90", "45", "15", "1"})
        n342 = local read "Snap to foot"() -> (w906:bool)
        n343 = Unbundle(w891) -> ("Hover Object"=w892:T14)  [unwired: 2 out]
        n344 = case shown="\"Down\"" w900 {
          tunnel: [cluster{dbl, dbl} {0.0, 0.0} ("Coord (ft)") cluster{dbl, dbl} {0.0, 0.1} ("Coord (ft)") cluster{dbl, dbl} {0.0, -0.1} ("Coord (ft)") cluster{dbl, dbl} {-0.1, 0.0} ("Coord (ft)") cluster{dbl, dbl} {0.1, 0.0} ("Coord (ft)")] -> w902
          tunnel: [_ w920 w922 w924 w926] -> w898
          tunnel: TRUE ("Delta") -> [_ w920 w922 w924 w926]
          frame Default {
          }
          frame "Up" {
          }
          frame "Down" {
          }
          frame "Left" {
          }
          frame "Right" {
          }
        }
        n345 = Unbundle(w892) -> ("Index"=w890:i32, "Pt Test Results"=w899:enum16{"Miss", "Rect Hit", "Arrow Hit"})
        n346 = Bundle("Snap robot to baseline"=w907, "Snap to foot"=w906, "Angle Limiter"=w905) -> (w904:T47)  [unwired: 1 in]
        n347 = case shown="\"Rect Hit\", Default" w899 {
          tunnel: [w910 w918] -> w908
          tunnel: w895 -> [_ w917]
          tunnel: w904 -> [_ w916]
          tunnel: w893 -> [w910 w915]
          tunnel: TRUE ("Delta") -> [_ w914]
          tunnel: w902 -> [_ w913]
          tunnel: w898 -> [_ w912]
          tunnel: [_ w912] -> w897
          tunnel: w890 -> [_ w911]
          frame "Miss" {
          }
          frame "Rect Hit", Default {
            n348 = call "Handle Pos and Rot.vi"("Delta"=w914, "Picture in"=w917, "Option"=w916, "Coord (ft)"=w913, "Index"=w911, "Points in"=w915) -> ("Points out"=w918:cluster{"x":dbl, "y":dbl, "th":dbl}[])  [unwired: 5 in]
          }
        }
        n349 = event-data("Discard?"=w897) -> ()  [unwired: 1 in, 1 out]
      }
      event User Event {
        n350 = event-data() -> ("Data"=w940:i32)  [unwired: 1 in]
        n351 = Unbundle(w933) -> ("Updated Waypoints"=w932:cluster{"x":dbl, "y":dbl, "th":dbl}[])  [unwired: 3 out]
        n352 = Tick Count (ms)() -> (millisecond timer value=w943:u32)
        n353 = Subtract(x=w943, y=w940) -> (x-y=w942:u32)
        n354 = Multiply(x=w942, y=0.001) -> (x*y=w939:dbl)
        n355 = local read "Duration (s)"() -> (w945:dbl)
        n356 = Quotient & Remainder(x=w939, y=0.02) -> (floor(x/y)=w937:dbl)  [unwired: 1 out]
        n357 = Multiply(x=0.02, y=w937) -> (x*y=w936:dbl)
        n358 = Less Or Equal?(x=w936, y=w945) -> (x <= y?=w946:bool)
        n359 = case shown="True" w946 {
          tunnel: w947 -> [_ w951]
          tunnel: w940 -> [_ w949]
          tunnel: w936 -> [_ w950]
          frame False {
          }
          frame True {
            n360 = local write "Time (s)"(w950) -> ()
            n361 = Generate User Event(user event=w951, event data cluster=w949) -> ()  [unwired: 2 in, 2 out]
          }
        }
        n362 = Wait (ms)(milliseconds to wait=u32 50) -> ()  [unwired: 1 out]
      }
      event "Tab Control": Value Change {
        n363 = event-data() -> ("NewVal"=w956:T6)  [unwired: 1 in]
        n364 = Unbundle(w959) -> ("Updated Waypoints"=w958:cluster{"x":dbl, "y":dbl, "th":dbl}[])  [unwired: 3 out]
        n365 = case shown="\"Command Sequencer\"" w956 {
          tunnel: [w962 w963] -> w955
          tunnel: w954 -> [w962 _]
          frame "Trajectory Settings", Default {
          }
          frame "Command Sequencer" {
            n366 = call "Find RT Projects.vi"() -> ("Targets"=w963:refnum<vi>[], "Project Names"=w964:string[])  [unwired: 10 in]
            n367 = property on="Projects" class="Ring (strict)"("Strings []"=w964) -> ()  [unwired: 2 in, 2 out]
          }
        }
      }
      event "Refresh": Value Change {
        # "Later make this load from file so it doesn't need to be recomputed so often"
        n368 = event-data() -> ()  [unwired: 1 in, 1 out]
        n369 = Unbundle(w978) -> ("Updated Waypoints"=w977:cluster{"x":dbl, "y":dbl, "th":dbl}[])  [unwired: 3 out]
        n370 = Index Array(array=w975, index="Projects") -> (element=w973:refnum<vi>)
        n371 = call "Find Command Names.vi"("TargetItem in"=w973) -> ("Paths"=w972:path[], "Command Info"=w971:T50)  [unwired: 9 in]
        n372 = call "Format Commands to Tree.vi"("Paths"=w972, "Command Info"=w971) -> ("2D Picture"=w970:picture, "Filtered Command Info Out"=w967:T2)  [unwired: 8 in]
        n373 = call "Resize Icons.vi"("Scale Factor"="Scale Factor", "Filtered Command Info Out"=w967) -> ("Filtered Command Info Out"=w966:T2)  [unwired: 9 in]
        n374 = local write "Command Palette"(w970) -> ()
        n375 = Bundle("Filtered Command Info Out"=w966, "2D Picture"=w970) -> (w969:T5)  [unwired: 1 in]
        n376 = local write "Cache"(w969) -> ()
      }
      event event #0x53 {
        n377 = event-data() -> ("AppRef"=w986:refnum<vi>, "VIName"=w988:string, "VIAppRef"=w984:refnum<vi>)  [unwired: 1 in, 1 out]
        n378 = Unbundle(w998) -> ("Updated Waypoints"=w997:cluster{"x":dbl, "y":dbl, "th":dbl}[])  [unwired: 3 out]
        n379 = Unbundle(w996) -> ("Filename"=w987:string)  [unwired: 2 out]
        n380 = property class="App"(reference=w986) -> ("App.Name"=w985:string)  [unwired: 1 in, 2 out]
        n381 = property class="App"(reference=w984) -> ("App.Name"=w983:string)  [unwired: 1 in, 2 out]
        n382 = Search and Replace String(input string=w987, search string=w988, replace string=w988) -> (number of replacements=w993:i32)  [unwired: 5 in, 3 out]
        n383 = call "Find Command with Tag.vi"("Command Tag"=w987, "Commands"=w982) -> ("Index"=w994:i32, "Found Command"=w995:cluster{"Time (s)":dbl, T3, bool}, "Found"=w991:bool)  [unwired: 7 in]
        n384 = Not Equal To 0?(x=w993) -> (x != 0?=w992:bool)
        n385 = And(x=w991, y=w992) -> (x .and. y?=w990:bool)
        n386 = case shown="True" w990 {
          tunnel: w995 -> [_ w1008]
          tunnel: w994 -> [_ w1015]
          tunnel: w982 -> [w1002 w1017]
          tunnel: [w1002 w1016] -> _
          tunnel: [_ FALSE] -> w989
          tunnel: w985 -> [_ _]
          tunnel: w983 -> [_ _]
          frame False {
          }
          frame True {
            n387 = Unbundle(w1008) -> (w1010:T3)  [unwired: 2 out]
            n388 = Unbundle(w1010) -> ("Path"=w1014:path)  [unwired: 6 out]
            n389 = Open VI Reference(vi path=w1014) -> (vi reference=w1012:refnum<vi>)  [unwired: 5 in, 1 out]
            n390 = property class="VI"(reference=w1012) -> (reference out=w1005:refnum<vi>, "Panel"=w1013:refnum<vi>)  [unwired: 1 in, 1 out]
            n391 = property class="Pnl"(reference=w1013) -> ("Controls[]"=w1011:refnum<vi>[])  [unwired: 1 in, 2 out]
            n392 = for {
              tunnel: w1011 -> [w1022] mode=indexing
              tunnel: [w1019] -> w1009 mode=indexing
              shift-right: [w1018] -> w1004
              shift-left: w1005 -> [w1018]
              n393 = property class="Ctl"(reference=w1022) -> ("Label.Text"=w1021:string, "Value"=w1020:variant)  [unwired: 1 in, 2 out]
              n394 = Bundle("Label.Text"=w1021, "Value"=w1020) -> (w1019:cluster{"Label.Text":string, "Value":variant})  [unwired: 1 in]
            }
            n395 = Bundle(cluster=w1010, "All Control Values Variant"=w1009) -> (w1007:T3)  [unwired: 6 in]
            n396 = Bundle(cluster=w1008, w1007) -> (w1006:cluster{"Time (s)":dbl, T3, bool})  [unwired: 2 in]
            n397 = Replace Array Subset(array=w1017, new element=w1006, index=w1015) -> (w1016:cluster{"Time (s)":dbl, T3, bool}[])
            n398 = Close Reference(reference=w1004) -> ()  [unwired: 1 in, 1 out]
          }
        }
      }
      event "Inhale": Value Change {
        n399 = event-data() -> ()  [unwired: 1 in, 1 out]
        n400 = Unbundle(w1033) -> ("Updated Waypoints"=w1032:cluster{"x":dbl, "y":dbl, "th":dbl}[])  [unwired: 3 out]
        n401 = Unbundle(w1031) -> ("Filename"=w1030:string)  [unwired: 2 out]
        n402 = call "Find Command with Tag.vi"("Command Tag"=w1030, "Commands"=w1025) -> ("Index"=w1027:i32, "Found Command"=w1028:cluster{"Time (s)":dbl, T3, bool}, "Found"=w1029:bool)  [unwired: 7 in]
        n403 = case shown="True" w1029 {
          tunnel: w1028 -> [_ w1046]
          tunnel: w1027 -> [_ w1053]
          tunnel: w1025 -> [w1037 w1055]
          tunnel: [w1037 w1054] -> w1026
          tunnel: [_ TRUE] -> w1024
          frame False {
          }
          frame True {
            n404 = Unbundle(w1046) -> (w1048:T3)  [unwired: 2 out]
            n405 = Unbundle(w1048) -> ("Path"=w1052:path)  [unwired: 6 out]
            n406 = Open VI Reference(vi path=w1052) -> (vi reference=w1050:refnum<vi>)  [unwired: 5 in, 1 out]
            n407 = property class="VI"(reference=w1050) -> (reference out=w1043:refnum<vi>, "Panel"=w1051:refnum<vi>)  [unwired: 1 in, 1 out]
            n408 = property class="Pnl"(reference=w1051) -> (reference out=w1041:refnum<vi>, "Controls[]"=w1049:refnum<vi>[])  [unwired: 1 in, 1 out]
            n409 = for {
              tunnel: w1049 -> [w1061] mode=indexing
              tunnel: [w1058] -> w1047 mode=indexing
              shift-right: [w1057] -> w1040
              shift-left: w1043 -> [w1057]
              shift-right: [w1056] -> _
              shift-left: w1041 -> [w1056]
              n410 = property class="Ctl"(reference=w1061) -> ("Label.Text"=w1060:string, "Value"=w1059:variant)  [unwired: 1 in, 2 out]
              n411 = Bundle("Label.Text"=w1060, "Value"=w1059) -> (w1058:cluster{"Label.Text":string, "Value":variant})  [unwired: 1 in]
            }
            n412 = Bundle(cluster=w1048, "All Control Values Variant"=w1047) -> (w1045:T3)  [unwired: 6 in]
            n413 = Bundle(cluster=w1046, w1045) -> (w1044:cluster{"Time (s)":dbl, T3, bool})  [unwired: 2 in]
            n414 = Replace Array Subset(array=w1055, new element=w1044, index=w1053) -> (w1054:cluster{"Time (s)":dbl, T3, bool}[])
            n415 = property class="VI"(reference=w1040, "FP.State"=T29."Closed" ("Front Panel Window:State")) -> (reference out=w1039:refnum<vi>)  [unwired: 1 in, 1 out]
            n416 = Close Reference(reference=w1039) -> ()  [unwired: 1 in, 1 out]
          }
        }
      }
      event "fps": Cursor Move {
        n417 = event-data() -> ("CursIdx"=w1064:i32, "CursLoc"=w1070:cluster{"X":dbl, "Y":dbl})  [unwired: 1 in]
        n418 = Unbundle(w1071) -> ("Updated Waypoints"=w1069:cluster{"x":dbl, "y":dbl, "th":dbl}[])  [unwired: 3 out]
        n419 = Array Size(array=w1067) -> (size(s)=w1066:i32)
        n420 = Greater?(x=w1066, y=w1064) -> (0:w1065:bool)
        n421 = case shown="False" w1065 {
          tunnel: w1070 -> [w1078 w1083]
          tunnel: w1067 -> [w1076 w1081]
          tunnel: [w1076 w1080] -> w1068
          tunnel: w1064 -> [_ w1079]
          frame False {
            n422 = Unbundle(w1078) -> ("X"=w1077:dbl)  [unwired: 1 out]
            n423 = local write "Time (s)"(w1077) -> ()
          }
          frame True {
            n424 = Unbundle(w1083) -> ("X"=w1082:dbl)  [unwired: 1 out]
            n425 = in-place {
              in-place-border: w1082 -> [w1086]
              n426 = in-place-array #2(w1081, w1079) -> (w1085:cluster{"Time (s)":dbl, T3, bool})
              n427 = Bundle(cluster=w1085, "Time (s)"=w1086) -> (w1084:cluster{"Time (s)":dbl, T3, bool})  [unwired: 2 in]
              n428 = in-place-array #2(w1084) -> (w1080:cluster{"Time (s)":dbl, T3, bool}[])  [unwired: 1 out]
            }
          }
        }
      }
      event "Command Sequence": Mouse Down {
        # "click on enable of row ?"
        n429 = event-data() -> ("CtlRef"=w1101:refnum<vi>, "Coords"=w1102:T45, "PlatMods.Shift"=w1087:bool)  [unwired: 1 in]
        n430 = Unbundle(w1104) -> ("Updated Waypoints"=w1103:cluster{"x":dbl, "y":dbl, "th":dbl}[])  [unwired: 3 out]
        n431 = invoke class="Tree (strict)" method="Point To Row Column"(reference=w1101, "Point"=w1102) -> ("Tag"=w1092:string, "Col"=w1096:i32)  [unwired: 6 in, 6 out]
        n432 = String Subset(string=w1092, length (rest)=2 ("length (rest)")) -> (substring=w1100:string)  [unwired: 1 in]
        n433 = Equal?(x=2 ("length (rest)"), y=w1096) -> (x = y?=w1095:bool)
        n434 = Equal?(x="//", y=w1100) -> (x = y?=w1094:bool)
        n435 = And(x=w1094, y=w1095) -> (x .and. y?=w1093:bool)
        n436 = case shown="True" w1093 {
          tunnel: w1091 -> [w1109 w1112]
          tunnel: w1092 -> [_ w1116]
          tunnel: [w1109 w1111] -> w1089
          tunnel: [_ TRUE] -> w1090
          tunnel: w1087 -> [_ w1110]
          frame False {
          }
          frame True {
            n437 = call "Find Command with Tag.vi"("Command Tag"=w1116, "Commands"=w1112) -> ("Index"=w1113:i32, "Found Command"=w1114:cluster{"Time (s)":dbl, T3, bool}, "Found"=w1115:bool)  [unwired: 7 in]
            n438 = case shown="False" w1110 {
              tunnel: w1115 -> [w1122 _]
              tunnel: w1114 -> [w1121 _]
              tunnel: w1113 -> [w1120 w1131]
              tunnel: w1112 -> [w1119 w1134]
              tunnel: [w1118 w1133] -> w1111
              frame False {
                # "Toggle"
                n439 = case shown="True" w1122 {
                  tunnel: w1121 -> [_ w1125]
                  tunnel: w1120 -> [_ w1128]
                  tunnel: w1119 -> [w1123 w1129]
                  tunnel: [w1123 w1126] -> w1118
                  frame False {
                  }
                  frame True {
                    n440 = Unbundle(w1125) -> (w1124:bool)  [unwired: 2 out]
                    n441 = Not(x=w1124) -> (.not. x?=w1130:bool)
                    n442 = Bundle(cluster=w1125, w1130) -> (w1127:cluster{"Time (s)":dbl, T3, bool})  [unwired: 2 in]
                    n443 = Replace Array Subset(array=w1129, new element=w1127, index=w1128) -> (w1126:cluster{"Time (s)":dbl, T3, bool}[])
                  }
                }
              }
              frame True {
                # "Delete"
                n444 = Delete From Array(array=w1134, length=1, index=w1131) -> (array with subset deleted=w1133:cluster{"Time (s)":dbl, T3, bool}[])  [unwired: 1 out]
              }
            }
          }
        }
      }
      event "Command Sequence": Double Click {
        n445 = event-data() -> ("CtlRef"=w1149:refnum<vi>, "Coords"=w1150:T45)  [unwired: 1 in]
        n446 = Unbundle(w1152) -> ("Updated Waypoints"=w1151:cluster{"x":dbl, "y":dbl, "th":dbl}[])  [unwired: 3 out]
        n447 = invoke class="Tree (strict)" method="Point To Row Column"(reference=w1149, "Point"=w1150) -> ("Tag"=w1139:string, "Col"=w1144:i32)  [unwired: 6 in, 6 out]
        n448 = String Subset(string=w1139, length (rest)=2 ("length (rest)")) -> (substring=w1148:string)  [unwired: 1 in]
        n449 = Equal?(x=0 ("length (rest)"), y=w1144) -> (x = y?=w1143:bool)
        n450 = Equal?(x="//", y=w1148) -> (x = y?=w1142:bool)
        n451 = And(x=w1142, y=w1143) -> (x .and. y?=w1141:bool)
        n452 = case shown="True" w1141 {
          tunnel: w1140 -> [_ w1160]
          tunnel: w1139 -> [_ w1158]
          tunnel: [_ w1157] -> w1136
          frame False {
          }
          frame True {
            n453 = call "Open Command Panel.vi"("Commands"=w1160, "Tag"=w1158) -> ("Found"=w1159:bool)  [unwired: 9 in]
            n454 = Select(t=w1158, s=w1159, f="") -> (s? t:f=w1157:string)
          }
        }
        n455 = Bundle(cluster=w1137, "Filename"=w1136) -> (w1138:T15)  [unwired: 2 in]
      }
      event "Command Sequence": Edit Cell? {
        n456 = event-data() -> ("String"=w1168:string, "Tag"=w1167:string, "Col"=w1170:i32)  [unwired: 1 in, 2 out]
        n457 = Unbundle(w1177) -> ("Updated Waypoints"=w1176:cluster{"x":dbl, "y":dbl, "th":dbl}[])  [unwired: 3 out]
        n458 = Equal?(x=1 ("length (rest)"), y=w1170) -> (x = y?=w1171:bool)
        n459 = String Subset(string=w1167, length (rest)=2 ("length (rest)")) -> (substring=w1175:string)  [unwired: 1 in]
        n460 = Equal?(x="//", y=w1175) -> (x = y?=w1172:bool)
        n461 = And(x=w1172, y=w1171) -> (x .and. y?=w1169:bool)
        n462 = case shown="True" w1169 {
          tunnel: [TRUE _] -> w1162
          tunnel: w1168 -> [_ w1191]
          tunnel: w1164 -> [w1182 w1188]
          tunnel: w1167 -> [_ w1187]
          tunnel: [w1182 w1189] -> w1165
          frame False {
          }
          frame True {
            n463 = call "Find Command with Tag.vi"("Command Tag"=w1187, "Commands"=w1188) -> ("Index"=w1185:i32, "Found Command"=w1184:cluster{"Time (s)":dbl, T3, bool}, "Found"=w1186:bool)  [unwired: 7 in]
            n464 = Scan From String(input string=w1191) -> (output 1=w1190:dbl)  [unwired: 4 in, 3 out]
            n465 = case shown="True" w1186 {
              tunnel: w1188 -> [w1192 w1195]
              tunnel: [w1192 w1196] -> w1189
              tunnel: w1190 -> [_ w1197]
              tunnel: w1185 -> [_ w1193]
              tunnel: w1184 -> [_ w1198]
              frame False {
              }
              frame True {
                n466 = Bundle(cluster=w1198, "Time (s)"=w1197) -> (w1194:cluster{"Time (s)":dbl, T3, bool})  [unwired: 2 in]
                n467 = Replace Array Subset(array=w1195, new element=w1194, index=w1193) -> (w1196:cluster{"Time (s)":dbl, T3, bool}[])
              }
            }
          }
        }
        n468 = event-data("Discard?"=w1162) -> ()  [unwired: 1 in, 1 out]
        n469 = Not(x=w1162) -> (.not. x?=w1163:bool)
      }
      event "Command Palette": Mouse Move {
        n470 = event-data() -> ("Coords"=w1206:T45)  [unwired: 1 in]
        n471 = Unbundle(w1209) -> ("Updated Waypoints"=w1208:cluster{"x":dbl, "y":dbl, "th":dbl}[])  [unwired: 3 out]
        n472 = control-ref of="Command Palette"() -> (w1202:refnum<vi>)
        n473 = Unbundle(w1199) -> ("Filtered Command Info Out"=w1204:T2, "2D Picture"=w1207:picture)
        n474 = call "Picture Coord to Row.vi"("Row Height"=w1201, "Coords"=w1206, "Picture in"=w1202) -> ("Row Index"=w1203:i32, "Clicked in canvas"=w1205:bool)  [unwired: 7 in]
        n475 = case shown="True" w1205 {
          tunnel: w1207 -> [_ w1217]
          tunnel: w1204 -> [_ _]
          tunnel: w1201 -> [_ w1215]
          tunnel: w1203 -> [_ w1214]
          frame False {
          }
          frame True {
            n476 = Multiply(x=w1214, y=w1215) -> (x*y=w1220:i32)
            n477 = Add(x=w1220, y=w1215) -> (x+y=w1221:i32)
            n478 = Bundle(0, w1220, 300, w1221) -> (w1222:cluster{i32, i32, i32, i32})  [unwired: 1 in]
            n479 = call <vilib>:"Draw Rectangle.vi"("rect"=w1222, "fill?(F)"=TRUE, "color(black)"=u32 10539263) -> ("new picture"=w1224:picture)  [unwired: 6 in]
            n480 = Concatenate Strings(w1224, w1217) -> (→"Command Palette":picture)
          }
        }
      }
      event "Command Palette": Mouse Down {
        n481 = event-data() -> ("Coords"=w1236:T45, "Mods"=w1238:cluster{"Double Click":bool, "Menu Key":bool})  [unwired: 1 in, 1 out]
        n482 = control-ref of="Command Palette"() -> (w1237:refnum<vi>)
        n483 = Unbundle(w1240) -> ("Updated Waypoints"=w1239:cluster{"x":dbl, "y":dbl, "th":dbl}[])  [unwired: 3 out]
        n484 = call "Picture Coord to Row.vi"("Row Height"=w1235, "Coords"=w1236, "Picture in"=w1237) -> ("Row Index"=w1231:i32, "Clicked in canvas"=w1234:bool)  [unwired: 7 in]
        n485 = Unbundle(w1238) -> ("Double Click"=w1233:bool)  [unwired: 1 out]
        n486 = Unbundle(w1226) -> ("Filtered Command Info Out"=w1230:T2)  [unwired: 1 out]
        n487 = Compound Arithmetic op=AND(w1234, w1233) -> (w1232:bool)
        n488 = case shown="True" w1232 {
          tunnel: w1231 -> [_ w1253]
          tunnel: w1230 -> [_ w1254]
          tunnel: w1228 -> [w1245 w1249]
          tunnel: [w1245 w1246] -> w1229
          frame False {
          }
          frame True {
            n489 = local read "Time (s)"() -> (w1250:dbl)
            n490 = Index Array(array=w1254, index=w1253) -> (element=w1252:T3)
            n491 = for {
              tunnel: w1249 -> [w1259] mode=indexing
              tunnel: w1250 -> [w1257]
              tunnel: [w1255] -> w1247
              i -> [w1255]
              stop <- w1256 stop-if-true
              n492 = Unbundle(w1259) -> ("Time (s)"=w1258:dbl)  [unwired: 2 out]
              n493 = Greater Or Equal?(x=w1258, y=w1257) -> (x >= y?=w1256:bool)
            }
            n494 = Bundle("Time (s)"=w1250, w1252, TRUE) -> (w1248:cluster{"Time (s)":dbl, T3, bool})  [unwired: 1 in]
            n495 = Insert Into Array(array=w1249, index=w1247, new element=w1248) -> (w1246:cluster{"Time (s)":dbl, T3, bool}[])
          }
        }
      }
    }
    n496 = feedback-in #1(w86) -> ()
    n497 = Unbundle(w52) -> ("Cluster 2"=w51:T30)  [unwired: 3 out]
    n498 = Unbundle(w51) -> ("Limits"=w53:T8)  [unwired: 3 out]
    n499 = Unbundle(w53) -> ("Velocity (fps)"=w50:dbl)  [unwired: 3 out]
    n500 = flat-sequence {
      tunnel: ["Time (s)"] -> w105
      tunnel: ["Sample Period (s)"] -> w69
      tunnel: ["Limits"] -> w40
      tunnel: ["Conditions"] -> w41
      tunnel: [w118] -> w58
      tunnel: ["Overrides"] -> w44
      tunnel: w62 -> [w118]
      tunnel: w61 -> [w117]
      tunnel: ["Hide Path"] -> w48
      tunnel: ["Stoopid Overlap %"] -> w47
      frame #0 {
        n501 = control-ref of="Command Sequence"() -> (w119:refnum<vi>)
        n502 = global write "Globals.vi" "> 90?"("Allow Angles > 90") -> ()
        n503 = call "Format Tree.vi"("Update"=w117, "Commands"=w118, "Tree Refnum"=w119) -> ()  [unwired: 9 in]
      }
    }
    n504 = control-ref of="Overrides"() -> (w45:refnum<vi>)
    n505 = Unbundle(w40) -> ("Accel (fps^2)"=w39:dbl)  [unwired: 3 out]
    n506 = Divide(x=w105, y=w69) -> (x/y=w96:dbl)
    n507 = Bundle("Sample Period (s)"=w69, "Limits"=w40, "Conditions"=w41, "Overrides"=w44) -> (w42:T30)  [unwired: 1 in]
    n508 = call "Enforce Robot Rules.vi"("max V"=w50, "Overrides"=w45, "turn accel"=w39, "Disable"=w97, "New Points"=w99, "Original Points"=w98) -> ("Points out"=w83:cluster{"x":dbl, "y":dbl, "th":dbl}[])  [unwired: 5 in]
    "WayPoints" <- w83
    n509 = call "GenNewTraj.vi"("Stoopid Overlap %"=w47, "Parameters"=w42, "Points in"=w83) -> ("Time (s)"=w87:dbl, "Valid"=w70:bool, "Trajectory Data"=w82:T1, "Updated Waypoints"=w88:cluster{"x":dbl, "y":dbl, "th":dbl}[], "Distance (ft)"=w89:dbl)  [unwired: 4 in]
    "Duration (s)" <- w87
    "Distance (ft)" <- w89
    "Trajectory Data" <- w82
    n510 = property on="Time (s)" class="Slide (strict)"("Scale.Minimum"=0.0 ("Scale.Range:Minimum"), "Scale.Maximum"=w87) -> ()  [unwired: 2 in, 2 out]
    n511 = Bundle("Time (s)"=w87, "Distance (ft)"=w89) -> (w101:cluster{"Time (s)":dbl, "Distance (ft)":dbl})  [unwired: 1 in]
    n512 = Bundle("Trajectory Data"=w82, "Updated Waypoints"=w88, w42, w58) -> (w43:T51)  [unwired: 1 in]
    n513 = call "Draw Trajectory.vi"("Robot Index"=w96, "Hide Path"=w48, "new picture in"=picture data[5B] ("new picture"), "Trajectory Data"=w82, "Picture in"=w108) -> ("Path Points"=w90:cluster{"x":dbl, "y":dbl}[], "Output Point"=w104:T52, "new picture"=w106:picture)  [unwired: 4 in]
    n514 = Unbundle(w80) -> ("Hover Object"=w79:T14)  [unwired: 2 out]
    n515 = call "Draw Shapes.vi"("Path Points"=w90, "Sample Period (s)"=w69, "Output Point"=w104, "Commands"=w58, "Results"=w79, "new picture in"=w106, "Points"=w88, "Picture in"=w108) -> ("new picture out"=→"Picture":picture)  [unwired: 3 in]
    n516 = call "Saved Checker.vi"("comp A"=w91, "comp B"=w43) -> ("Unsaved"=w54:bool)
    n517 = call "Update Annotations.vi"("Sample Period"=w69, "Commands"=w58, "Trajectory Data"=w82, "Robot Pt Index"=w96) -> ("Redraw"=w60:bool, "Velocity Trace"=w59:dbl[], "Annotation Data"=w95:T53)  [unwired: 5 in]
    n518 = Select(t=0, s=w74, f=2000) -> (s? t:f=w75:i32)
    n519 = Select(t=cluster{u32, u32}[] [{14869218, 14869218}] ("Colors [4]"), s=w70, f=cluster{u32, u32}[] [{6094681, 6094681}] ("Colors [4]")) -> (s? t:f=w73:cluster{u32, u32}[])
    n520 = case shown="True" w60 {
      tunnel: w95 -> [_ w112]
      tunnel: w59 -> [_ w111]
      frame False {
      }
      frame True {
        n521 = property on="fps" class="WFGraph (strict)"("AnntList"=w112) -> ()  [unwired: 2 in, 2 out]
        "fps" <- w111
      }
    }
    n522 = Select(t=u32 16711680 ("Boolean Text.Text Colors:Text Color"), s=w54, f=u32 0 ("Boolean Text.Text Colors:Text Color")) -> (s? t:f=w55:u32)
    n523 = property on="Unjank" class="Bool"("Colors [4]"=w73) -> ()  [unwired: 2 in, 2 out]
    n524 = property on="Save" class="Bool"("BoolText.TextColor"=w55) -> ()  [unwired: 2 in, 2 out]
  }
  n525 = Format Into String(format string=w18, w3) -> (resulting string=w19:string)  [unwired: 2 in, 1 out]
  n526 = property class="VI"("Front Panel.Title"=w19) -> ()  [unwired: 2 in, 2 out]
